vi "WHD_VEten_0.1.3_WS_BIDIR_Calibr.vi"() -> ()   [LabVIEW 2015]
uses:
  <vilib>/NI_Real-Time Target Support.lvlib
  <vilib>/rvi/interface/nirviReadWriteControl/nirviReadWriteControl.xnode
  <vilib>/rvi/interface/nirviMethod/nirviMethod.xnode
  <vilib>/rvi/interface/nirviOpenFPGA/nirviOpenFPGA.xnode
  <vilib>/rvi/interface/nirviCloseFPGA/nirviCloseFPGA.xnode
  <vilib>/userDefined/High Color/nirio_resource_hc.ctl
  <vilib>/rvi/errors/niLvFpgaMergeErrorWithErrorCode.vi
  <vilib>/Utility/file.llb/Write Delimited Spreadsheet (string).vi
  <vilib>/RTwatchdog.llb/Watchdog expiration actions.ctl
  <vilib>/nisyscfg/nisyscfg.lvlib
  AURA_Wheel/Json2Labv.lvlib
  AURA_Wheel/AuraWheelAPI/AuraWheel.lvlib
  <vilib>/rvi/errors/niLvFpgaAdjustHostInterfaceError.vi
  NiFpgaLv.dll
  <vilib>/Utility/error.llb/Error Cluster From Error Code.vi
  <vilib>/LabVIEW Targets/FPGA/cRIO/shared/nicrio_ModuleControls/nicrio_cRIO-9234_DataRatesRing2.ctl
  <vilib>/FPGAPlugInAG/cRIO-9031/niLvFpga_Run_cRIO-9031.vi
  <vilib>/FPGAPlugInAG/cRIO-9031/niLvFpga_ConfigureFifo_cRIO-9031.vi
  <vilib>/FPGAPlugInAG/cRIO-9031/niLvFpga_StartFifo_cRIO-9031.vi
  <vilib>/FPGAPlugInAG/cRIO-9031/niLvFpga_ReadFifo_cRIO-9031.vi
  <vilib>/FPGAPlugInAG/cRIO-9031/niLvFpga_StopFifo_cRIO-9031.vi
  <vilib>/FPGAPlugInAG/cRIO-9031/niLvFpga_Reset_cRIO-9031.vi
  <vilib>/measure/NI_MAPro.lvlib
  <vilib>/Analysis/NI_AALPro.lvlib
  <vilib>/measure/maspectr.llb/FFT Spectrum (Mag-Phase) for 1 Chan.vi
  <vilib>/Analysis/5stat.llb/RMS (DBL).vi
  <vilib>/measure/madcrms.llb/Basic Averaged DC-RMS for 1 Chan.vi
  FPGA Bitfiles/W&RDArabia_FPGATarget_FPGA8a2wsBIdirec_yJvL9yuTbZw.lvbitx
  <vilib>/FPGAPlugInAG/cRIO-9031/niLvFpga_Open_cRIO-9031.vi
  <vilib>/FPGAPlugInAG/cRIO-9031/niLvFpga_Close_cRIO-9031.vi
panel:
  in  "LR6 IP address":string="192.168.106.94"
  in  "Port LR6":u16=2001
  out "T fuera rango":bool
  in  "Frecuencia de muestreo (Hz)":dbl=25600.0
  in  "Escaneos de la FIFO por canal":u32=5000
  in  "Tiempo extra al detector de paso (s)":dbl=1.0
  in  "dt RMS":dbl=256.0
  in  "Frecuencia de muestreo y módulo CRIO":T1=2 items=["51.200 kS/s (NI 9234)"=1, "25.600 kS/s (NI 9234)"=2, "17.067 kS/s (NI 9234)"=3, "12.800 kS/s (NI 9234)"=4, "10.240 kS/s (NI 9234)"=5, "8.533 kS/s (NI 9234)"=6, "7.314 kS/s (NI 9234)"=7, "6.400 kS/s (NI 9234)"=8, "5.689 kS/s (NI 9234)"=9, "5.120 kS/s (NI 9234)"=10, "4.654 kS/s (NI 9234)"=11, "4.267 kS/s (NI 9234)"=12, "3.938 kS/s (NI 9234)"=13, "3.657 kS/s (NI 9234)"=14, "3.413 kS/s (NI 9234)"=15, "3.200 kS/s (NI 9234)"=16, "3.012 kS/s (NI 9234)"=17, "2.845 kS/s (NI 9234)"=18, "2.695 kS/s (NI 9234)"=19, "2.560 kS/s (NI 9234)"=20, "2.438 kS/s (NI 9234)"=21, "2.328 kS/s (NI 9234)"=22, "2.226 kS/s (NI 9234)"=23, "2.133 kS/s (NI 9234)"=24, "2.048 kS/s (NI 9234)"=25, "1.969 kS/s (NI 9234)"=26, "1.896 kS/s (NI 9234)"=27, "1.829 kS/s (NI 9234)"=28, "1.765 kS/s (NI 9234)"=29, "1.707 kS/s (NI 9234)"=30, "1.652 kS/s (NI 9234)"=31]
  in  "Puerto RFID":u16=2189
  in  "IP RFID":string="192.168.106.99"
  in  "Offset_rueda WS 2":fxp<+/-,24,-4>=0.004999998956918716 format="%.27g"
  in  "Count(mSec)":u32=2
  in  "RFID NEM on?":bool
  in  "RFID LR6 on?":bool
  in  "Canal cero WS1?":bool
  in  "Canal cero WS2":bool
  out "Inicio pasada 2":timestamp
  in  "Calibration":bool
  out "Direccion 0?":bool
  out "Boton Adquirir?":bool
  out "RuedaDetectada2?":bool=TRUE
  out "RuedaDetectada1?":bool=TRUE
  in  "Timeout ruedas":dbl
  in  "Borrar archivos\nadquisicion con error":bool
  in  "Able watchdog?":bool
  in  "Reset watchdog?":bool
  in  "Leer config RFID NEM":bool
  in  "bytes to read":i32
  in  "DeviceAddress":u8
  in  "timeout ms (60000)":i32
  in  "Max archivos":u32=2
  in  "Bytes libre despues de borrar":u32=2
  in  "Bytes min libre":u32=2
  in  "Nº de acelerómetros":i32
  in  "Nº inductivos":i32
  in  "Offset_rueda WS 1":fxp<+/-,24,-4>=0.004999998956918716 format="%.27g"
  out "TAGs_AURAwheel":string[][](array[string])
  out "Plataformas?":bool
  out "Nº Ejes":i32[](array[numeric])
  out "Nº UTs":i32
  out "it-read-LR6":i32[](array[numeric])
  out "it-LR6":i32
  out "RFID_LR6_Error":errorcluster
  out "Series_flota":string[](array[string])
  out "Tabla_flota":string[][](array[string])
  out "Puntos medios de las ventanas":dbl[][](array[numeric])
  out "configuration file path":path=path "c:/Parametros.cfg"
  in  "IP synchr":string
  out "data":cluster{"status":string}
  out "confRFID":path=path "c:/RFID/TAGS.csv"
  out "TAGS leidos":path=path "c:/RFID/TAGS.csv"
  in  "Use Aura?":bool
  in  "Parametros AuraWheel":string[](array[string])
  in  "Parámetros acelerómetros":dbl[](array[numeric])
  out "Fin":bool
  out "Contador":i32=1
  out "Path TEST":path=path "c:/TEST"
  out "Fallo fotocelula":bool
  out "Path_Borrar":path=path "c:/Trenes"
  out "Longitud de la unidad":dbl
  out "Aviso no detección":string
  out "Time to Acquire Block (ms)":i32
  out "Distancia de acelerómetros":dbl[](array[numeric])
  out "Block Size":u32
  out "Distancias generales":dbl[](array[numeric])
  in  "Reset del controlador":bool
  in  "Configuración":bool
  in  "Parar la aplicación":bool
  out "RFID":bool=TRUE
  out "date/time string":string
  out "Timeout ruedas":bool
  out "Tiempo":dbl
  out "Inicio pasada":timestamp
  out "Ultimo TEST":timestamp
  out "Fuente":bool=TRUE
  out "Estado":string
  out "RFID_ID":refnum<k5>
  out "DC OK":string
  out "Aviso temperatura":string
  in  "Tab Control":T2(tab)=enum."Datos adquisición"
  out "String":string
  out "V (m/s)":dbl
  out "Temperatura (ºC)":dbl
  out "Max RMS Ruedas":dbl[][](array[numeric])
  out "result":bool
  out "TAGs":string[](array[string])
  out "Parar":bool
  out "TAGs LR6":string[](array[string])
  out "TAGs HEX":string[](array[string])
  out "Waveform Graph 2":sgl[](graph)
  out "Waveform Graph":sgl[][](graph)
  out "Nombre de archivo":path[](array[path])
  out "Tiempo de paso (s)":dbl
  out "Tiempo extra de adquisición (s)":dbl
  out "Número de ejes detectados":i32
  out "Buffer Underflow":bool
  out "Buffer Overflow":bool
  out "Disco Duro Disponible (bytes)":i64
  out "created path":path
  out "Nº Ruedas 1":i32
  out "NºRuedas 2":i32
  out "deleted portion":sgl[](array[numeric])
  out "deleted portion 2":sgl[](array[numeric])
  out "Ejes_convoy":i32
  out "Archivo\nvalido?":bool
  out "Parámetros":bool=TRUE
  out "Distacias y medidas de dispositivos":bool=TRUE
  out "RFID_Error":errorcluster
  out "error FPGA":errorcluster
  out "error manipulacion archivos":errorcluster
  out "Unidades y ejes":bool=TRUE
  out "RFID":bool=TRUE
  out "error AURA":errorcluster
  out "Response headers":string
  out "Numeric 3":i32
  in  "Digital?":bool=TRUE
  out "Bucle Espera":i32
  out "Watchdog config":T3={"reset"=FALSE, "occurrence"=FALSE, "trigger protocol"=enum."active high", "trigger line"=enum."none", "disable watchdog on VI exit"=TRUE}
  out "error out":errorcluster
  in  "stop":bool
  in  "Tiempo de adquisicion":dbl=10.0
  in  "Adquirir":bool
  out "Waveform Graph 4":waveform(dbl)[](graph)
  out "Waveform Graph 3":cluster{"f0":dbl, "df":dbl, "magnitude":dbl[]}(graph)
  out "Chassis \nTemperature":i16
  out "Frecuencia de excitación\nVibrómetro  (Hz)":dbl
  out "Tiempo de paso (s) 2":dbl
  out "Nombre de archivo 2":path
  out "Buffer Overflow 2":bool
  out "Buffer Underflow 2":bool
  in  "Adquirir 2":bool
  in  "Nº del canal":i32
  in  "Parámetro de sensibilidad\n           (mV/g)":sgl=10.0
  in  "Aceleración del patrón (g RMS)":dbl=1.0
  in  "Frecuencia del patrón (Hz)":dbl=159.2
  # "Funciona?"
  # "Última detección de unidad"
  # "Error!!"
  # "Estado de la memoria"
  # "Cargar datos de configuración"
  # "Errores!!"
  # "WRD_MEX\nWRD_ZAR"
  # "0 tagMexInit\n1 tagMexFin\n\n0 tag1\n1 tag2"
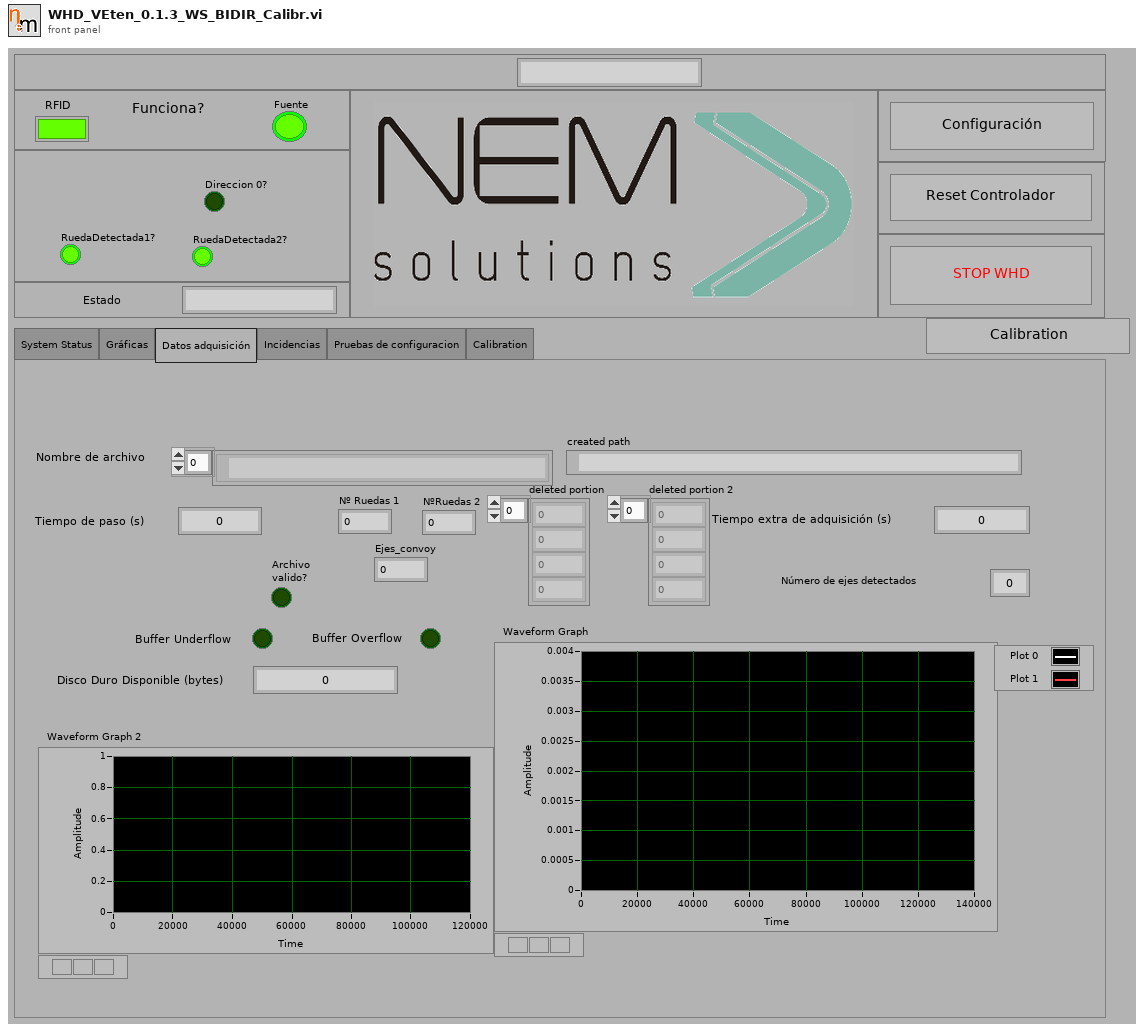
[diagram p1: front panel]
types:
  T1 = typedef "nicrio_cRIO-9234_DataRatesRing2.ctl" = u8
  T2 = enum32{"System Status", "Gráficas", "Datos adquisición", "Incidencias", "Pruebas de configuracion", "Calibration"}
  T3 = typedef "Watchdog expiration actions.ctl" = cluster{"reset":bool, "occurrence":bool, "trigger protocol":enum16{"active high", "active low", "open collector"}, "trigger line":enum16{"none", "line 0", "line 1", "line 2", "line 3", "line 4", "line 5", "line 6", "line 7", "SMB line 0"}, "disable watchdog on VI exit":bool}
  T4 = typedef "nirio_resource_hc.ctl" = tag
  T5 = enum16{"Standard", "Buffered", "CRLF", "Immediate"}
  T6 = enum16{"open", "replace", "create", "open or create", "replace or create", "replace or create with confirmation"}
  T7 = enum16{"big-endian, network order", "native, host order", "little-endian"}
  T8 = cluster{"error IO":errorcluster, bool[], u32[], string[], dbl[]}
  T9 = cluster{"g_ts":dbl, "p_sp":dbl, "p_tp":dbl, "p_tg":cluster{"tg_n":dbl, "tg_t":string}[], "p_ax":cluster{"ax_n":dbl, "ax_sp":dbl, "ax_wh":cluster{"wh_p":dbl, "wh_a1":dbl, "wh_a2":dbl, "wh_a3":dbl, "wh_a4":dbl}[]}[]}
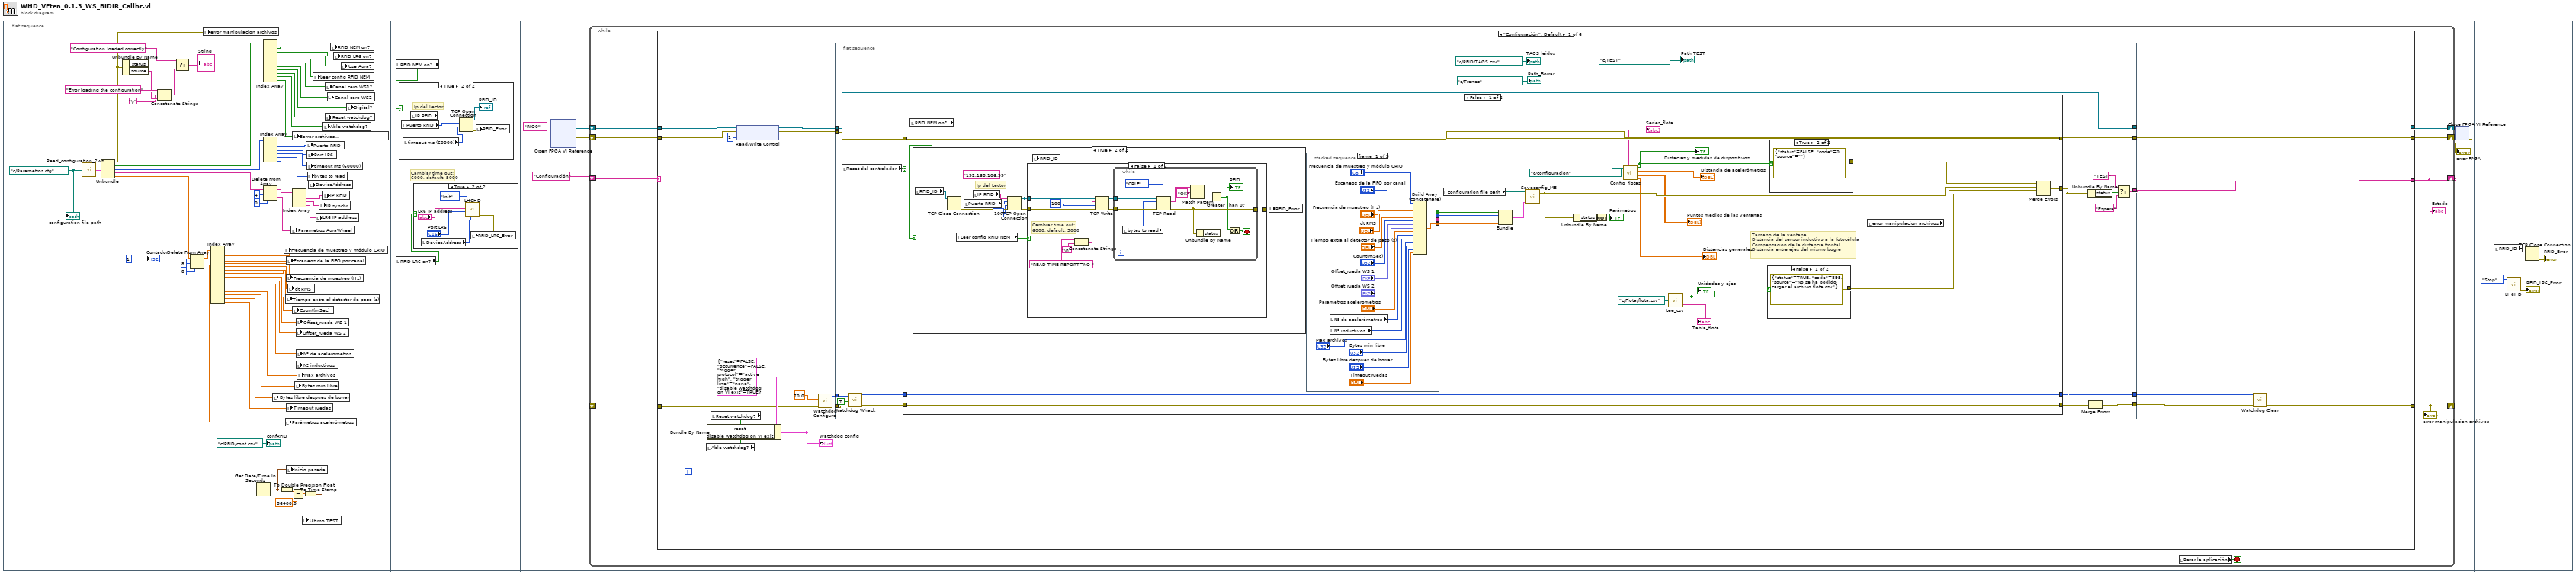
[diagram p0: block diagram]
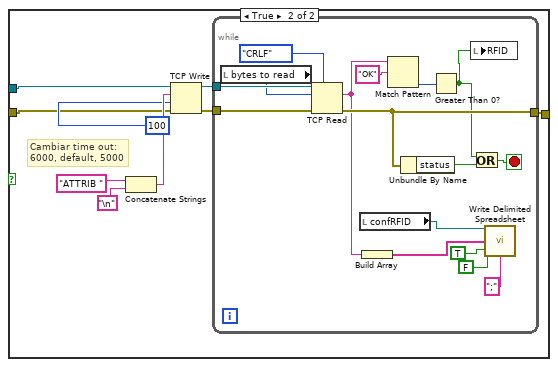
[diagram p5: hidden frame]
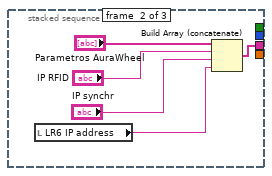
[diagram p6: hidden frame]
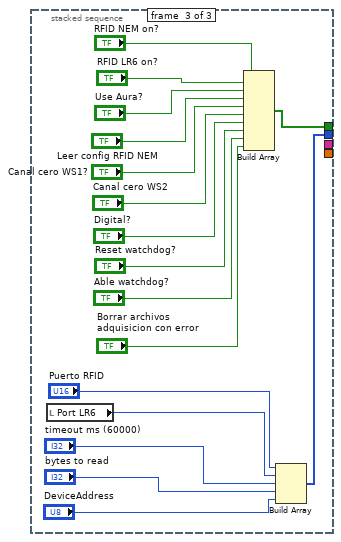
[diagram p7: hidden frame]
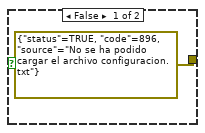
[diagram p8: hidden frame]
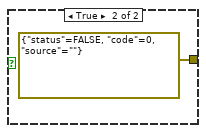
[diagram p9: hidden frame]
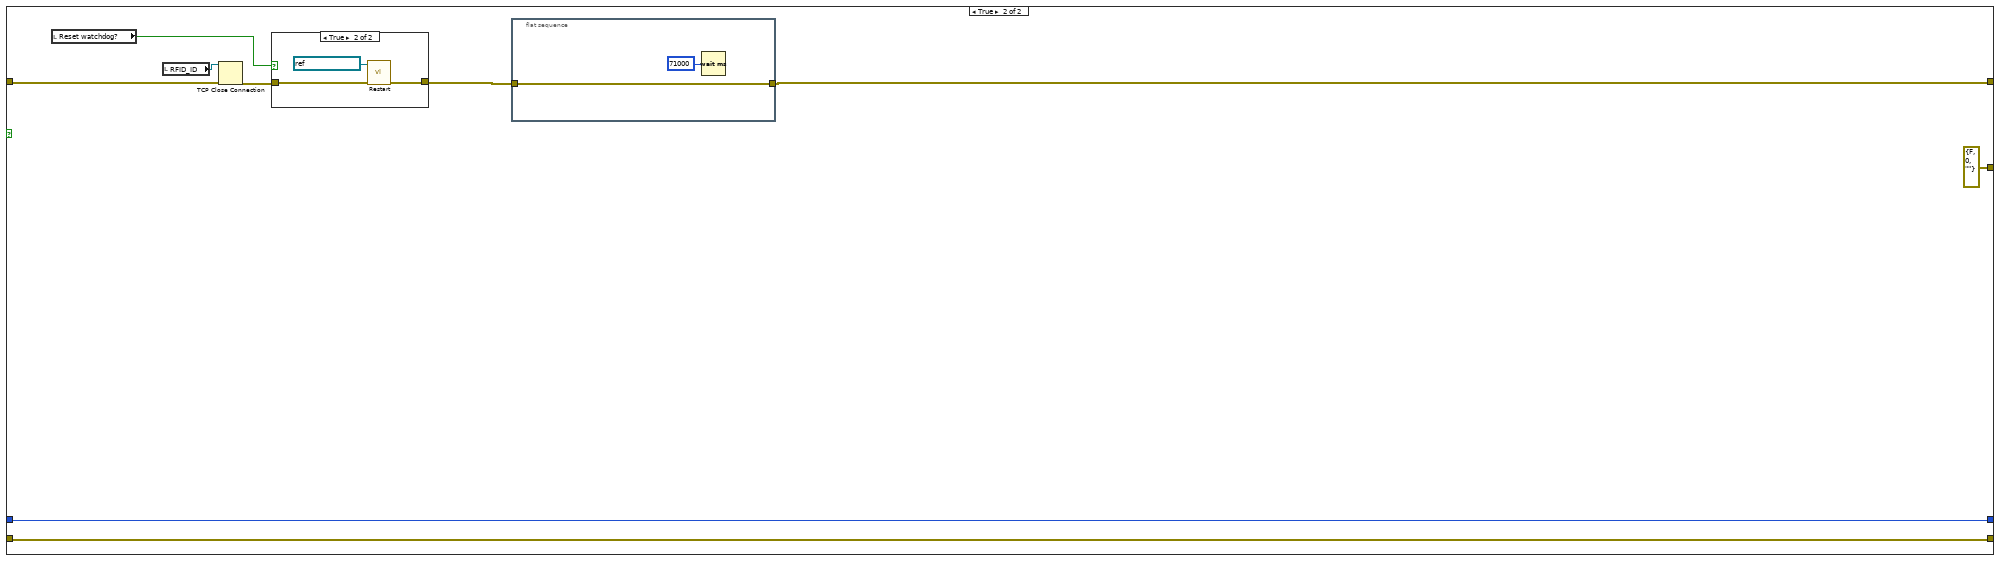
[diagram p10: hidden frame]
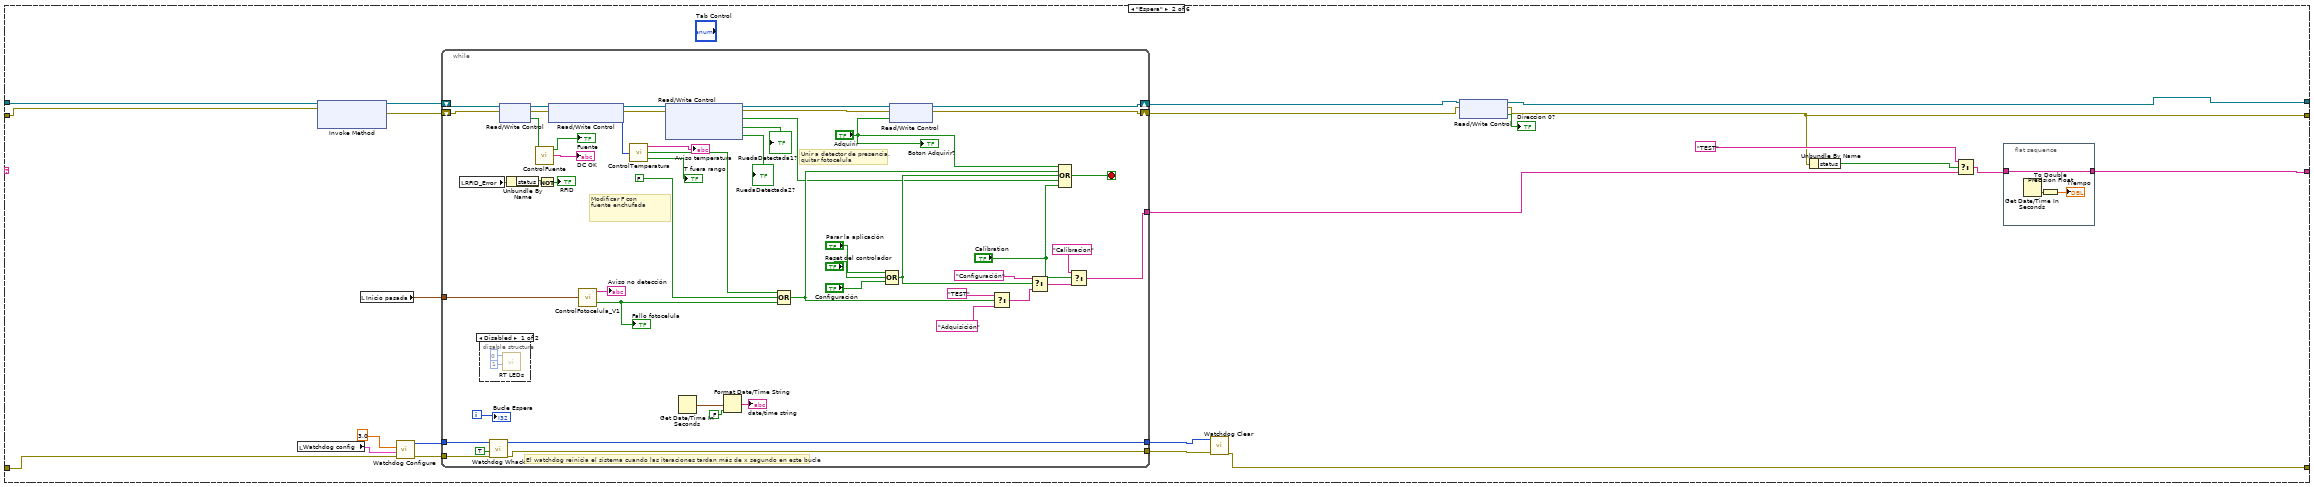
[diagram p12: hidden frame]
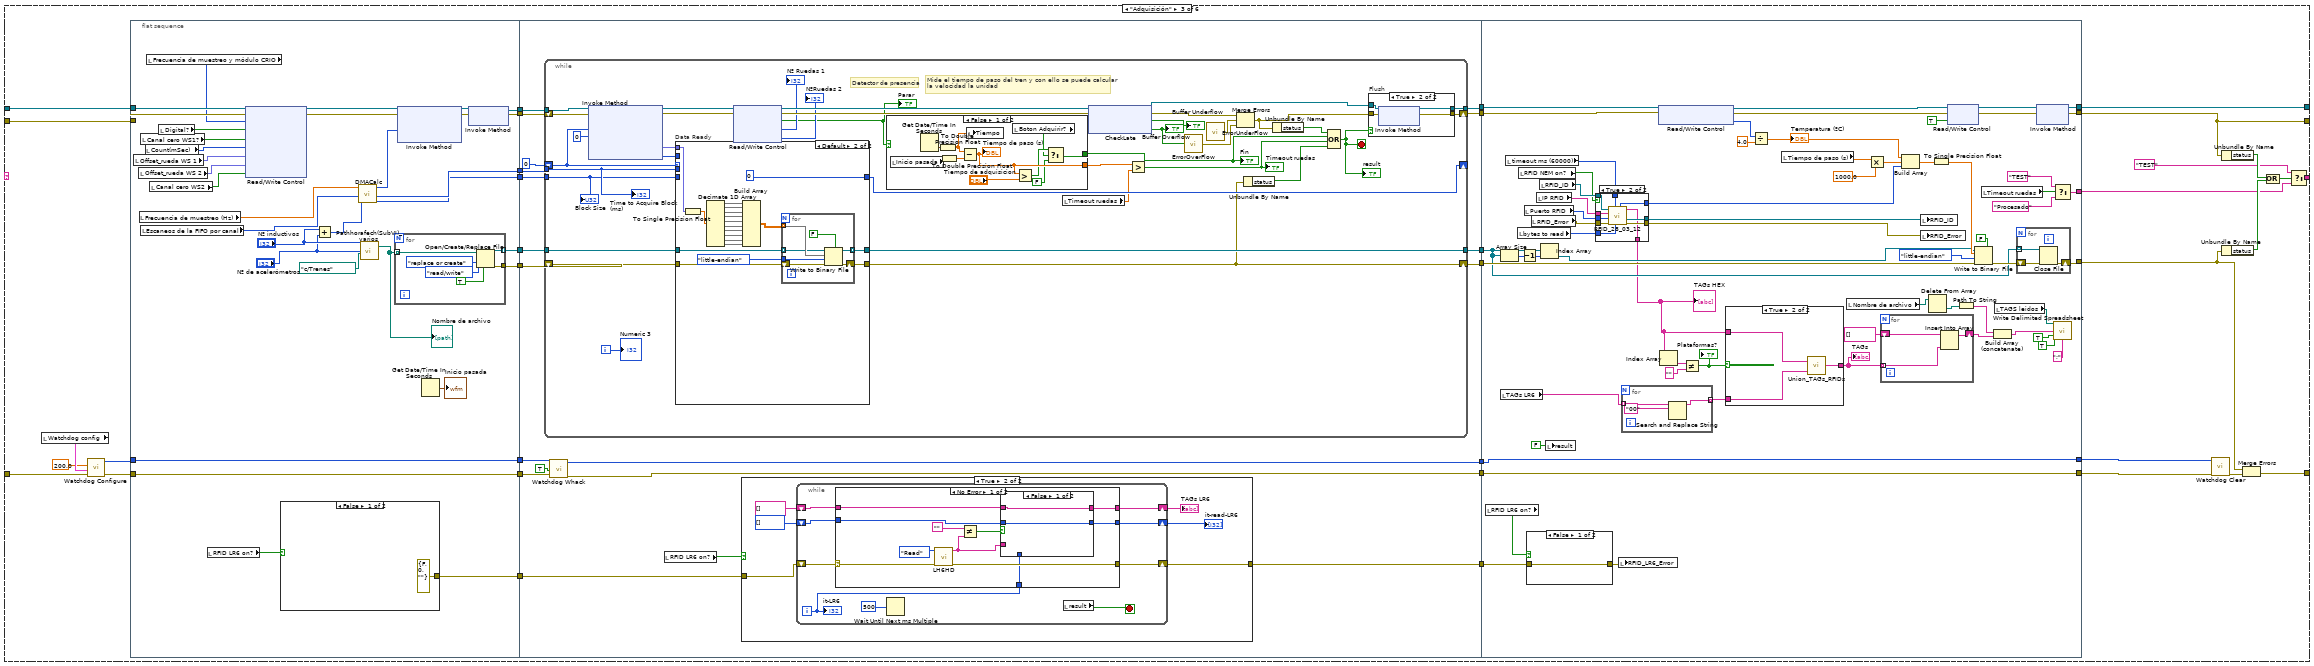
[diagram p14: hidden frame]
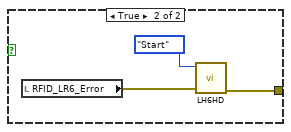
[diagram p15: hidden frame]
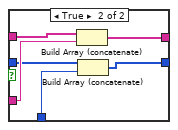
[diagram p17: hidden frame]
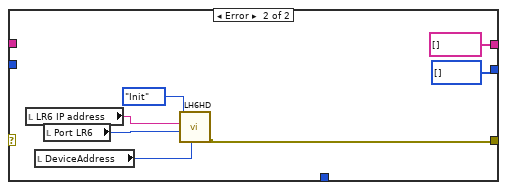
[diagram p18: hidden frame]
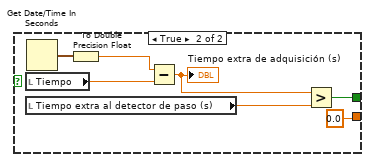
[diagram p19: hidden frame]
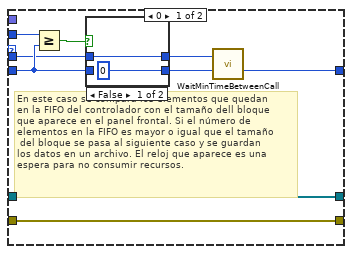
[diagram p20: hidden frame]
diagram:
  n1 = flat-sequence {
    frame #0 {
      w46 = path "c:/Parametros.cfg" ("configuration file path")
      n2 = call "Read_configuration_2ws.vi"("configuration file path"=w46) -> ("output cluster"=w45:T8)
      n3 = Unbundle(w45) -> ("error IO"=w8:errorcluster, w49:bool[], w48:u32[], w37:string[], w43:dbl[])
      n4 = Unbundle By Name(w8) -> ("status"=w7:bool, "source"=w4:string)
      n5 = Concatenate Strings("Error loading the configuration", "\r", w4) -> (w2:string)
      n6 = Select(t="Configuration loaded correctly", s=w7, f=w2) -> (s? t:f=→"String":string)
      n7 = Delete From Array(array=w43, length=8, index=8) -> (deleted portion=w39:dbl[], array with subset deleted=w42:dbl[])
      n8 = local write "error manipulacion archivos"(w8) -> ()
      n9 = Index Array(array=w42) -> (element #1=w56:dbl, element #2=w55:dbl, element #3=w54:dbl, element #4=w53:dbl, element #5=w52:dbl, element #6=w27:dbl, element #7=w26:dbl, element #8=w9:dbl, element #9=w25:dbl, element #10=w24:dbl, element #11=w23:dbl, element #12=w22:dbl, element #13=w21:dbl, element #14=w10:dbl)  [unwired: 14 in]
      n10 = Get Date/Time In Seconds() -> (seconds since 1Jan1904=w58:timestamp)
      n11 = Index Array(array=w49) -> (element #1=w51:bool, element #2=w50:bool, element #3=w38:bool, element #4=w17:bool, element #5=w16:bool, element #6=w15:bool, element #7=w14:bool, element #8=w13:bool, element #9=w12:bool, element #10=w11:bool)  [unwired: 10 in]
      n12 = Index Array(array=w48) -> (element #1=w44:u32, element #2=w28:u32, element #3=w20:u32, element #4=w19:u32, element #5=w18:u32)  [unwired: 5 in]
      n13 = Delete From Array(array=w37, length=4, index=0) -> (deleted portion=w31:string[], array with subset deleted=w36:string[])
      n14 = local write "Bytes libre despues de borrar"(w21) -> ()
      n15 = To Double Precision Float(number=w58) -> (double precision float=w60:dbl)
      n16 = local write "Frecuencia de muestreo y módulo CRIO"(w56) -> ()
      n17 = local write "Parámetros acelerómetros"(w39) -> ()
      n18 = local write "Tiempo extra al detector de paso (s)"(w52) -> ()
      n19 = local write "Frecuencia de muestreo (Hz)"(w54) -> ()
      n20 = local write "Timeout ruedas"(w10) -> ()
      n21 = local write "Escaneos de la FIFO por canal"(w55) -> ()
      n22 = local write "Inicio pasada"(w58) -> ()
      n23 = local write "dt RMS"(w53) -> ()
      n24 = local write "Parametros AuraWheel"(w31) -> ()
      n25 = Subtract(x=w60, y=86400.0) -> (x-y=w59:dbl)
      n26 = local write "Borrar archivos\nadquisicion con error"(w11) -> ()
      n27 = Index Array(array=w36) -> (element #1=w30:string, element #2=w32:string, element #3=w29:string)  [unwired: 3 in]
      n28 = local write "Count(mSec)"(w27) -> ()
      n29 = local write "Bytes min libre"(w22) -> ()
      n30 = local write "Offset_rueda WS 2"(w9) -> ()
      n31 = local write "Offset_rueda WS 1"(w26) -> ()
      n32 = local write "Nº de acelerómetros"(w25) -> ()
      n33 = local write "Nº inductivos"(w24) -> ()
      n34 = local write "Max archivos"(w23) -> ()
      n35 = To Time Stamp(1:w59) -> (0:w57:timestamp)
      n36 = local write "Ultimo TEST"(w57) -> ()
      n37 = local write "Puerto RFID"(w44) -> ()
      n38 = local write "Port LR6"(w28) -> ()
      n39 = local write "timeout ms (60000)"(w20) -> ()
      n40 = local write "bytes to read"(w19) -> ()
      n41 = local write "DeviceAddress"(w18) -> ()
      n42 = local write "Leer config RFID NEM"(w17) -> ()
      n43 = local write "LR6 IP address"(w29) -> ()
      n44 = local write "IP synchr"(w32) -> ()
      n45 = local write "IP RFID"(w30) -> ()
      n46 = local write "Able watchdog?"(w12) -> ()
      n47 = local write "Reset watchdog?"(w13) -> ()
      n48 = local write "Canal cero WS1?"(w16) -> ()
      n49 = local write "Canal cero WS2"(w15) -> ()
      n50 = local write "RFID NEM on?"(w51) -> ()
      n51 = local write "RFID LR6 on?"(w50) -> ()
      n52 = local write "Use Aura?"(w38) -> ()
      n53 = local write "Digital?"(w14) -> ()
      "Contador" <- 1
      "confRFID" <- path "c:/RFID/conf.csv" ("file path (use dialog)")
      "configuration file path" <- w46
    }
    frame #1 {
      # "Cambiar time out:\n6000, default, 5000"
      n54 = local read "RFID NEM on?"() -> (w63:bool)
      n55 = local read "RFID LR6 on?"() -> (w62:bool)
      n56 = case shown="True" w63 {
        frame False {
        }
        frame True {
          # "Ip del Lector"
          n57 = local read "Puerto RFID"() -> (w71:u16)
          n58 = local read "timeout ms (60000)"() -> (w69:i32)
          n59 = local read "IP RFID"() -> (w72:string)
          n60 = TCP Open Connection(address=w72, remote port or service name=w71, timeout ms (60000)=w69) -> (connection ID=→"RFID_ID":refnum<k5>, error out=w70:errorcluster)  [unwired: 1 in, 1 out]
          n61 = local write "RFID_Error"(w70) -> ()
        }
      }
      n62 = case shown="True" w62 {
        frame False {
        }
        frame True {
          n63 = local read "DeviceAddress"() -> (w64:u8)
          n64 = call "LH6HD.vi"("DeviceAddress"=w64, "Reader Port"="Port LR6", "IP Address"="LR6 IP address", "Action"=enum16{"Init", "Start", "Read", "Stop", "Exit"}."Init") -> ("error out"=w68:errorcluster)  [unwired: 6 in, 1 out]
          n65 = local write "RFID_LR6_Error"(w68) -> ()
        }
      }
    }
    frame #2 {
      n66 = xnode "Open FPGA VI Reference"("resource name"=T4 "RIO0") -> ("FPGA VI Reference Out"=w80:refnum<k20>, "error out"=w79:errorcluster)  [unwired: 1 in]
      n67 = while {
        shift-right: [w81] -> _
        shift-left: "Configuración" -> [w89]
        shift-right: [w83] -> w76
        shift-left: w80 -> [w88]
        shift-right: [w82] -> w75
        shift-left: w79 -> [w87]
        shift-right: [w86] -> _
        shift-left: _ -> [w85]
        stop <- w84 stop-if-true
        n68 = case shown="\"Configuración\", Default" w89 {
          tunnel: [w95 w279 w358 w689 w930 _] -> w81
          tunnel: [w107 w267 w372 w697 w929 _] -> w83
          tunnel: [w108 w266 w373 w684 w927 _] -> w82
          tunnel: w88 -> [w100 w284 w380 w697 w929 w1002]
          tunnel: w87 -> [w98 w282 w379 w684 w928 w1001]
          tunnel: [w104 w273 w370 w687 w917 _] -> w86
          tunnel: w85 -> [w94 w278 w354 w683 w922 _]
          frame "Configuración", Default {
            n69 = local read "Able watchdog?"() -> (w101:bool)
            n70 = local read "Reset watchdog?"() -> (w102:bool)
            n71 = Bundle By Name(cluster=T3 {"reset"=FALSE, "occurrence"=FALSE, "trigger protocol"=enum."active high", "trigger line"=enum."none", "disable watchdog on VI exit"=TRUE} ("expiration actions"), "reset"=w102, "disable watchdog on VI exit"=w101) -> (w93:T3)
            "Watchdog config" <- w93
            n72 = xnode "Read/Write Control"("FPGA VI Reference In"=w100, "error in"=w98, "Cycles to Filter"=u16 1) -> ("FPGA VI Reference Out"=w99:refnum<k20>, "error out"=w97:errorcluster)
            n73 = call <vilib>:"Watchdog Configure.vi"("error in (no error)"=w94, "expiration actions"=w93, "timeout (1 sec)"=70.0) -> ("error out"=w90:errorcluster, "watchdogID"=w91:u64)  [unwired: 1 in, 2 out]
            n74 = flat-sequence {
              tunnel: [w119] -> w108
              tunnel: [w127] -> w95
              tunnel: w99 -> [w120]
              tunnel: [w120] -> w107
              tunnel: [w122] -> w105
              tunnel: w97 -> [w117]
              tunnel: [w114] -> w106
              tunnel: w91 -> [w110]
              tunnel: w90 -> [w109]
              frame #0 {
                n75 = local read "Reset del controlador"() -> (w116:bool)
                n76 = call <vilib>:"Watchdog Whack.vi"("error in (no error)"=w109, "reset watchdog after expire? (F)"=TRUE, "watchdogID in"=w110) -> ("error out"=w112:errorcluster, "watchdogID out"=w113:u64)  [unwired: 2 in, 1 out]
                n77 = case shown="False" w116 {
                  tunnel: w117 -> [w154 w257]
                  tunnel: [w154 w256] -> w119
                  tunnel: [w140 errorcluster {"status"=FALSE, "code"=0, "source"=""} ("error IO")] -> w118
                  tunnel: [w132 w255] -> w114
                  tunnel: w113 -> [w132 w255]
                  tunnel: w112 -> [w131 w254]
                  tunnel: [w131 w254] -> w111
                  frame False {
                    # "Tamaño de la ventana\nDistancia del sensor inductivo a la fotocélula\nCompensación de la distancia frontal\nDistancia entre ejes del mismo bogie"
                    n78 = local read "RFID NEM on?"() -> (w130:bool)
                    n79 = case shown="True" w130 {
                      frame False {
                      }
                      frame True {
                        (unwired) "192.168.106.99" ("address")
                        # "Ip del Lector"
                        n80 = local read "RFID_ID"() -> (w162:refnum<k5>)
                        n81 = TCP Close Connection(connection ID=w162) -> (error out=w163:errorcluster)  [unwired: 2 in, 1 out]
                        n82 = local read "Leer config RFID NEM"() -> (w155:bool)
                        n83 = local read "Puerto RFID"() -> (w160:u16)
                        n84 = local read "IP RFID"() -> (w159:string)
                        n85 = TCP Open Connection(address=w159, remote port or service name=w160, timeout ms (60000)=100, error in (no error)=w163) -> (connection ID=w161:refnum<k5>, error out=w156:errorcluster)  [unwired: 1 out]
                        n86 = case shown="False" w155 {
                          tunnel: w161 -> [w172 w186]
                          tunnel: [w170 w184] -> w157
                          tunnel: w156 -> [w167 w185]
                          frame False {
                            # "Cambiar time out:\n6000, default, 5000"
                            n87 = Concatenate Strings("READ TIME REPORT=NO " ("data in"), "\n") -> (w164:string)
                            n88 = TCP Write(connection ID=w172, data in=w164, error in (no error)=w167, 9:100 ("timeout ms (25000)")) -> (connection ID out=w168:refnum<k5>, error out=w169:errorcluster)  [unwired: 1 out]
                            n89 = while {
                              tunnel: w169 -> [w182]
                              tunnel: w168 -> [w181]
                              tunnel: [w180] -> w170
                              stop <- w177 stop-if-true
                              n90 = local read "bytes to read"() -> (w173:i32)
                              n91 = TCP Read(connection ID=w181, bytes to read=w173, error in (no error)=w182, 7:T5."CRLF" ("mode (standard)")) -> (data out=w175:string, error out=w180:errorcluster)  [unwired: 1 in, 1 out]
                              n92 = Match Pattern(string=w175, regular expression="OK") -> (offset past match=w178:i32)  [unwired: 4 out]
                              n93 = Unbundle By Name(w180) -> ("status"=w176:bool)
                              n94 = Greater Than 0?(x=w178) -> (x > 0?=w174:bool)
                              "RFID" <- w174
                              n95 = Or(x=w174, y=w176) -> (x .or. y?=w177:bool)
                            }
                          }
                          frame True {
                            # "Cambiar time out:\n6000, default, 5000"
                            n96 = Concatenate Strings("ATTRIB " ("data in"), "\n") -> (w192:string)
                            n97 = TCP Write(connection ID=w186, data in=w192, error in (no error)=w185, 9:100 ("timeout ms (25000)")) -> (connection ID out=w189:refnum<k5>, error out=w188:errorcluster)  [unwired: 1 out]
                            n98 = while {
                              tunnel: w188 -> [w207]
                              tunnel: w189 -> [w206]
                              tunnel: [w205] -> w184
                              stop <- w202 stop-if-true
                              n99 = local read "bytes to read"() -> (w193:i32)
                              n100 = TCP Read(connection ID=w206, bytes to read=w193, error in (no error)=w207, 7:T5."CRLF" ("mode (standard)")) -> (data out=w196:string, error out=w205:errorcluster)  [unwired: 1 in, 1 out]
                              n101 = local read "confRFID"() -> (w195:path)
                              n102 = Build Array(w196) -> (w194:string[])
                              n103 = Match Pattern(string=w196, regular expression="OK") -> (offset past match=w203:i32)  [unwired: 4 out]
                              n104 = Unbundle By Name(w205) -> ("status"=w201:bool)
                              n105 = Greater Than 0?(x=w203) -> (x > 0?=w200:bool)
                              n106 = local write "RFID"(w200) -> ()
                              n107 = Or(x=w200, y=w201) -> (x .or. y?=w202:bool)
                              n108 = call-poly <vilib>:"Write Delimited Spreadsheet.vi"("file path (dialog if empty)"=w195, "1D data"=w194, "append to file? (F)"=FALSE ("transpose? (no:F)"), "transpose? (F)"=TRUE ("append to file? (new file:F)"), "delimiter (\\t)"=";" ("delimiter (\\t)")) -> ()  [unwired: 9 in, 2 out]
                            }
                          }
                        }
                        n109 = local write "RFID_ID"(w161) -> ()
                        n110 = local write "RFID_Error"(w157) -> ()
                      }
                    }
                    n111 = stacked-sequence {
                      tunnel: [w220 _ _] -> w144
                      tunnel: [_ w229 _] -> w143
                      tunnel: [_ _ w243] -> w145
                      tunnel: [_ _ w242] -> w146
                      frame #0 {
                        n112 = local read "Nº de acelerómetros"() -> (w214:i32)
                        n113 = local read "Nº inductivos"() -> (w213:i32)
                        n114 = Build Array (concatenate)("Frecuencia de muestreo y módulo CRIO", "Escaneos de la FIFO por canal", "Frecuencia de muestreo (Hz)", "dt RMS", "Tiempo extra al detector de paso (s)", "Count(mSec)", "Offset_rueda WS 1", "Offset_rueda WS 2", "Parámetros acelerómetros", w214, w213, "Max archivos", "Bytes min libre", "Bytes libre despues de borrar", "Timeout ruedas") -> (w220:dbl[])
                      }
                      frame #1 {
                        n115 = local read "LR6 IP address"() -> (w225:string)
                        n116 = Build Array (concatenate)("Parametros AuraWheel", "IP RFID", "IP synchr", w225) -> (w229:string[])
                      }
                      frame #2 {
                        n117 = local read "Port LR6"() -> (w239:u16)
                        n118 = Build Array("RFID NEM on?", "RFID LR6 on?", "Use Aura?", "Leer config RFID NEM", "Canal cero WS1?", "Canal cero WS2", "Digital?", "Reset watchdog?", "Able watchdog?", "Borrar archivos\nadquisicion con error") -> (w242:bool[])
                        n119 = Build Array("Puerto RFID", w239, "timeout ms (60000)", "bytes to read", "DeviceAddress") -> (w243:i32[])
                      }
                    }
                    n120 = local read "configuration file path"() -> (w141:path)
                    n121 = Bundle(w146, w145, w143, w144) -> (w142:cluster{bool[], i32[], string[], dbl[]})  [unwired: 1 in]
                    n122 = call "Saveconfig_MB.vi"("configuration file path"=w141, "Configuracion"=w142) -> ("error out"=w149:errorcluster)  [unwired: 4 in]
                    n123 = Unbundle By Name(w149) -> ("status"=w150:bool)
                    n124 = Not(x=w150) -> (.not. x?=→"Parámetros":bool)
                    n125 = call "Config_flotas.vi"("file path (dialog if empty)"=path "c:/configuracion") -> ("Distancias generales"=→"Distancias generales":dbl[], "Puntos medios de las ventanas"=→"Puntos medios de las ventanas":dbl[][], "Distancia de acelerómetros"=→"Distancia de acelerómetros":dbl[], "Distacias y medidas de dispositivos"=w139:bool, "Series_flota"=→"Series_flota":string[])  [unwired: 3 in]
                    "Distacias y medidas de dispositivos" <- w139
                    n126 = call "Lee_csv.vi"("Path"=path "c:/Flota/flota.csv") -> ("Tabla_flota"=→"Tabla_flota":string[][], "Lectura_OK?"=w136:bool)
                    "Unidades y ejes" <- w136
                    n127 = case shown="False" w136 {
                      tunnel: [errorcluster {"status"=TRUE, "code"=895, "source"="No se ha podido cargar el archivo flota.csv"} ("error out") errorcluster {"status"=FALSE, "code"=0, "source"=""} ("error out")] -> w147
                      frame False {
                      }
                      frame True {
                      }
                    }
                    n128 = case shown="True" w139 {
                      tunnel: [errorcluster {"status"=TRUE, "code"=896, "source"="No se ha podido cargar el archivo configuracion.txt"} ("error out") errorcluster {"status"=FALSE, "code"=0, "source"=""} ("error out")] -> w152
                      frame False {
                      }
                      frame True {
                      }
                    }
                    n129 = local read "error manipulacion archivos"() -> (w148:errorcluster)
                    n130 = Merge Errors(w152, w149, w148, w147) -> (w140:errorcluster)
                  }
                  frame True {
                    n131 = local read "Reset watchdog?"() -> (w251:bool)
                    n132 = local read "RFID_ID"() -> (w259:refnum<k5>)
                    n133 = TCP Close Connection(connection ID=w259, error in (no error)=w257) -> (error out=w253:errorcluster)  [unwired: 2 out]
                    n134 = case shown="True" w251 {
                      tunnel: w253 -> [w260 w263]
                      tunnel: [w260 w262] -> w252
                      frame False {
                      }
                      frame True {
                        n135 = call <vilib>:"Restart.vi"("error in (no error)"=w263, "Session in"=refnum<k21> "localhost") -> ("error out"=w262:errorcluster)  [unwired: 7 in, 2 out]
                      }
                    }
                    n136 = flat-sequence {
                      tunnel: [w265] -> w256
                      tunnel: w252 -> [w265]
                      frame #0 {
                        n137 = Wait (ms)(milliseconds to wait=u32 71000) -> ()  [unwired: 1 out]
                      }
                    }
                  }
                }
                n138 = Unbundle By Name(w118) -> ("status"=w128:bool)
                n139 = Merge Errors(w118, w111) -> (w122:errorcluster)
                n140 = Select(t="TEST", s=w128, f="Espera") -> (s? t:f=w127:string)
                "Path_Borrar" <- path "c:/Trenes" ("file path (use dialog)")
                "Path TEST" <- path "c:/TEST" ("file path (use dialog)")
                "TAGS leidos" <- path "c:/RFID/TAGS.csv" ("file path (use dialog)")
              }
            }
            n141 = call <vilib>:"Watchdog Clear.vi"("error in (no error)"=w105, "watchdogID in"=w106) -> ("error out"=w104:errorcluster)  [unwired: 5 in]
          }
          frame "Espera" {
            n142 = local read "Watchdog config"() -> (w272:T3)
            n143 = xnode "Invoke Method"("FPGA VI Reference In"=w284, "error in"=w282) -> ("FPGA VI Reference Out"=w283:refnum<k20>, "error out"=w281:errorcluster)  [unwired: 1 in]
            n144 = local read "Inicio pasada"() -> (w288:timestamp)
            n145 = call <vilib>:"Watchdog Configure.vi"("error in (no error)"=w278, "expiration actions"=w272, "timeout (1 sec)"=3.0) -> ("error out"=w277:errorcluster, "watchdogID"=w276:u64)  [unwired: 1 in, 2 out]
            n146 = while {
              tunnel: [w294] -> w287
              shift-right: [w304] -> w268
              shift-left: w283 -> [w317]
              shift-right: [w303] -> w269
              shift-left: w281 -> [w316]
              tunnel: w288 -> [w320]
              tunnel: w277 -> [w301]
              tunnel: w276 -> [w302]
              tunnel: [w300] -> w275
              tunnel: [w299] -> w274
              i -> [w297]
              stop <- w292 stop-if-true
              # "Modificar F con\nfuente enchufada"
              # "Unir a detector de presencia,\nquitar fotocelula"
              # "El watchdog reinicia el sistema cuando las iteraciones tardan más de x segundo en este bucle"
              n147 = local read "RFID_Error"() -> (w323:errorcluster)
              n148 = disable-structure shown="Disabled" {
                frame Disabled {
                  n149 = call <vilib>:"RT LEDs.vi"("State"=1, "LED Num"=0) -> ()  [unwired: 1 in, 5 out]
                }
                frame Enabled {
                }
              }
              n150 = call <vilib>:"Watchdog Whack.vi"("error in (no error)"=w301, "reset watchdog after expire? (F)"=TRUE, "watchdogID in"=w302) -> ("error out"=w299:errorcluster, "watchdogID out"=w300:u64)  [unwired: 2 in, 1 out]
              n151 = xnode "Read/Write Control"("FPGA VI Reference In"=w317, "error in"=w316) -> ("FPGA VI Reference Out"=w334:refnum<k20>, "error out"=w333:errorcluster, "DC OK"=w338:bool)
              n152 = Unbundle By Name(w323) -> ("status"=w321:bool)
              n153 = call "ControlFuente.vi"("DC OK 3"=w338) -> ("DC OK 2"=→"Fuente":bool, "DC OK"=→"DC OK":string)  [unwired: 1 out]
              n154 = Not(x=w321) -> (.not. x?=→"RFID":bool)
              n155 = xnode "Read/Write Control"("FPGA VI Reference In"=w334, "error in"=w333) -> ("FPGA VI Reference Out"=w329:refnum<k20>, "error out"=w328:errorcluster, "Chassis Temperature"=w336:i16)
              n156 = call "ControlFotocelula_V1.vi"("Tiempo de entrada a espera"=w320) -> ("Aviso no detección"=→"Aviso no detección":string, "Boolean"=w326:bool)
              "Fallo fotocelula" <- w326
              n157 = call "ControlTemperatura.vi"("Chassis Temperature"=w336) -> ("Aviso temperatura"=→"Aviso temperatura":string, "Boolean"=w330:bool, "T fuera rango"=→"T fuera rango":bool)
              n158 = xnode "Read/Write Control"("FPGA VI Reference In"=w329, "error in"=w328) -> ("FPGA VI Reference Out"=w319:refnum<k20>, "error out"=w318:errorcluster, "Detector de presencia"=w311:bool, "RuedaDetectada1?"=→"RuedaDetectada1?":bool, "RuedaDetectada2?"=→"RuedaDetectada2?":bool)
              n159 = Get Date/Time In Seconds() -> (seconds since 1Jan1904=w313:timestamp)
              n160 = Format Date/Time String(seconds (now)=w313, UTC format=FALSE) -> (date/time string=→"date/time string":string)  [unwired: 1 in]
              n161 = Compound Arithmetic op=OR(w330, FALSE ("value"), w326) -> (w327:bool)
              n162 = Compound Arithmetic op=OR("Parar la aplicación", "Reset del controlador", "Configuración") -> (w324:bool)
              n163 = xnode "Read/Write Control"("FPGA VI Reference In"=w319, "error in"=w318, "Fotocélula"="Adquirir") -> ("FPGA VI Reference Out"=w304:refnum<k20>, "error out"=w303:errorcluster)
              n164 = Select(t="TEST", s=w327, f="Adquisición") -> (s? t:f=w339:string)
              n165 = Select(t="Configuración", s=w324, f=w339) -> (s? t:f=w296:string)
              n166 = Compound Arithmetic op=OR("Adquirir", w327, w324, w311, "Calibration") -> (w292:bool)
              n167 = Select(t="Calibracion", s="Calibration", f=w296) -> (s? t:f=w294:string)
              "Bucle Espera" <- w297
              "Boton Adquirir?" <- "Adquirir"
            }
            n168 = call <vilib>:"Watchdog Clear.vi"("error in (no error)"=w274, "watchdogID in"=w275) -> ("error out"=w273:errorcluster)  [unwired: 5 in]
            n169 = xnode "Read/Write Control"("FPGA VI Reference In"=w268, "error in"=w269) -> ("FPGA VI Reference Out"=w267:refnum<k20>, "error out"=w266:errorcluster, "Direccion 0?"=→"Direccion 0?":bool)
            n170 = Unbundle By Name(w266) -> ("status"=w286:bool)
            n171 = Select(t="TEST", s=w286, f=w287) -> (s? t:f=w280:string)
            n172 = flat-sequence {
              tunnel: [w290] -> w279
              tunnel: w280 -> [w290]
              frame #0 {
                n173 = Get Date/Time In Seconds() -> (seconds since 1Jan1904=w291:timestamp)
                n174 = To Double Precision Float(number=w291) -> (double precision float=→"Tiempo":dbl)
              }
            }
          }
          frame "Adquisición" {
            n175 = local read "Watchdog config"() -> (w355:T3)
            n176 = call <vilib>:"Watchdog Configure.vi"("error in (no error)"=w354, "expiration actions"=w355, "timeout (1 sec)"=200.0) -> ("error out"=w352:errorcluster, "watchdogID"=w353:u64)  [unwired: 1 in, 2 out]
            n177 = flat-sequence {
              tunnel: w379 -> [w408]
              tunnel: w380 -> [w409]
              tunnel: [w407] -> w369
              tunnel: [w406] -> w368
              tunnel: [w405] -> w367
              tunnel: [w404] -> w366
              tunnel: [w403] -> w365
              tunnel: [w402] -> w364
              tunnel: [w391] -> w357
              tunnel: w353 -> [w390]
              tunnel: w352 -> [w389]
              tunnel: [w390] -> w351
              tunnel: [w389] -> w350
              tunnel: [w424] -> w378
              tunnel: [w441] -> w377
              tunnel: [w440] -> w376
              tunnel: [w439] -> w375
              tunnel: [w432] -> w374
              tunnel: w369 -> [w438]
              tunnel: w368 -> [w437]
              tunnel: w367 -> [w436]
              tunnel: w366 -> [w435]
              tunnel: w365 -> [w434]
              tunnel: w364 -> [w433]
              tunnel: w357 -> [w430]
              tunnel: [w429] -> w356
              tunnel: w351 -> [w428]
              tunnel: w350 -> [w427]
              tunnel: [w425] -> w349
              tunnel: w378 -> [w589]
              tunnel: w377 -> [w584]
              tunnel: w376 -> [w583]
              tunnel: w375 -> [w605]
              tunnel: [w635] -> w361
              tunnel: w374 -> [w637]
              tunnel: [w621] -> w371
              tunnel: [w622] -> w373
              tunnel: [w623] -> w372
              tunnel: w356 -> [w599]
              tunnel: w349 -> [w590]
              tunnel: [w590] -> w347
              tunnel: [w589] -> w346
              frame #0 {
                n178 = local read "Offset_rueda WS 1"() -> (w382:fxp<+/-,24,-4>)
                n179 = local read "Offset_rueda WS 2"() -> (w383:fxp<+/-,24,-4>)
                n180 = local read "Frecuencia de muestreo (Hz)"() -> (w400:dbl)
                n181 = local read "Escaneos de la FIFO por canal"() -> (w388:u32)
                n182 = local read "Canal cero WS1?"() -> (w393:bool)
                n183 = local read "Count(mSec)"() -> (w392:u32)
                n184 = local read "Frecuencia de muestreo y módulo CRIO"() -> (w395:T1)
                n185 = local read "Canal cero WS2"() -> (w381:bool)
                n186 = local read "Digital?"() -> (w394:bool)
                n187 = local read "RFID LR6 on?"() -> (w384:bool)
                n188 = xnode "Read/Write Control"("FPGA VI Reference In"=w409, "error in"=w408, "Data Rate"=w395, "Digital?"=w394, "Canal cero WS1?"=w393, "Count(mSec)"=w392, "Offset_WS1"=w382, "Offset_WS2"=w383, "Canal cero WS2?"=w381) -> ("FPGA VI Reference Out"=w399:refnum<k20>, "error out"=w398:errorcluster)
                n189 = case shown="False" w384 {
                  tunnel: [errorcluster {"status"=FALSE, "code"=0, "source"=""} ("error out") w414] -> w391
                  frame False {
                  }
                  frame True {
                    n190 = local read "RFID_LR6_Error"() -> (w415:errorcluster)
                    n191 = call "LH6HD.vi"("error in (no error)"=w415, "Action"=enum16{"Init", "Start", "Read", "Stop", "Exit"}."Start") -> ("error out"=w414:errorcluster)  [unwired: 8 in, 1 out]
                  }
                }
                n192 = Add(x="Nº inductivos", y="Nº de acelerómetros") -> (x+y=w386:i32)
                n193 = call "DMACalc.vi"("Number of Channels"=w386, "Number of Samples"=w388, "Rate (Hz)"=w400) -> ("Block Size"=w404:u32, "Time to Acquire Block (ms)"=w405:i32, "Host Buffer Size"=w410:u32)  [unwired: 6 in]
                n194 = call "Pathhorafech(SubVI)_varios.vi"("Folder path"=path "c:/Trenes", "Nº de acelerómetros"="Nº de acelerómetros", "Nº inductivos"="Nº inductivos") -> ("Acel_Paths"=w396:path[])  [unwired: 1 in, 1 out]
                "Nombre de archivo" <- w396
                n195 = for {
                  tunnel: w396 -> [w419] mode=indexing
                  tunnel: [w418] -> w403 mode=indexing
                  tunnel: [w417] -> w402
                  n196 = Open/Create/Replace File(file path (use dialog)=w419, operation (0:open)=T6."replace or create", access (0:read/write)=enum16{"read/write", "read-only", "write-only"}."read/write", disable buffering (F)=TRUE) -> (refnum out=w418:refnum<file>, error out=w417:errorcluster)  [unwired: 1 in, 2 out]
                }
                n197 = xnode "Invoke Method"("FPGA VI Reference In"=w399, "error in"=w398, "Requested Depth"=w410) -> ("FPGA VI Reference Out"=w412:refnum<k20>, "error out"=w411:errorcluster)  [unwired: 1 out]
                n198 = Get Date/Time In Seconds() -> (seconds since 1Jan1904=→"Inicio pasada":timestamp)
                n199 = xnode "Invoke Method"("FPGA VI Reference In"=w412, "error in"=w411) -> ("FPGA VI Reference Out"=w407:refnum<k20>, "error out"=w406:errorcluster)
              }
              frame #1 {
                n200 = while "Data Acquisition" {
                  tunnel: w438 -> [w493]
                  shift-right: [w518] -> _
                  shift-left: u32 0 ("t") -> [w514]
                  tunnel: w436 -> [w519]
                  tunnel: w435 -> [w517]
                  shift-right: [w520] -> w440
                  shift-left: w437 -> [w511]
                  tunnel: [w515] -> w441
                  tunnel: w434 -> [w497]
                  tunnel: [w498] -> w439
                  shift-right: [w496] -> w432
                  shift-left: w433 -> [w507]
                  i -> [w492]
                  stop <- w516 stop-if-true
                  # "Detector de presencia"
                  # "Mide el tiempo de paso del tren y con ello se puede calcular\nla velocidad la unidad"
                  n201 = xnode "Invoke Method"("FPGA VI Reference In"=w493, "error in"=w511, "Number of Elements"=w514, "Timeout (ms)"=0) -> ("FPGA VI Reference Out"=w489:refnum<k20>, "error out"=w495:errorcluster, "Data"=w510:fxp<+/-,24,4>[], "Elements Remaining"=w512:u32)
                  n202 = case "Data Ready" shown="Default" w514 {
                    tunnel: w519 -> [w542 _]
                    tunnel: [w541 u32 0 ("t")] -> w518
                    tunnel: w517 -> [w543 _]
                    tunnel: w512 -> [w540 _]
                    tunnel: w510 -> [_ w565]
                    tunnel: w507 -> [w539 w564]
                    tunnel: [w539 w566] -> w496
                    tunnel: w497 -> [w538 w563]
                    tunnel: [w538 w562] -> w498
                    frame 0 {
                      # "En este caso se compara los elementos que quedan\nen la FIFO del controlador con el tamaño dell bloque\nque aparece en el panel frontal. Si el número de \nelementos en la FIFO es mayor o igual que el tamaño\n del bloque se pasa al siguiente caso y se guardan \nlos datos en un archivo. El reloj que aparece es una\nespera para no consumir recursos."
                      n203 = Greater Or Equal?(x=w540, y=w543) -> (x >= y?=w544:bool)
                      n204 = case shown="False" w544 {
                        tunnel: [u32 0 ("Block Size") w548] -> w541
                        tunnel: [w547 0 ("t")] -> w545
                        tunnel: w542 -> [w547 _]
                        tunnel: w543 -> [_ w548]
                        frame False {
                        }
                        frame True {
                        }
                      }
                      n205 = call "WaitMinTimeBetweenCall.vi"("Minimum ms between calls"=w545) -> ()  [unwired: 2 in]
                    }
                    frame Default {
                      n206 = To Single Precision Float(number=w565) -> (single precision float=w552:sgl[])
                      n207 = Decimate 1D Array(w552) -> (w558:sgl[], w561:sgl[], w560:sgl[], w559:sgl[], w557:sgl[], w556:sgl[], w555:sgl[], w554:sgl[], w553:sgl[], w550:sgl[])
                      n208 = Build Array(w558, w561, w560, w559, w557, w556, w555, w554, w553, w550) -> (w551:sgl[][])
                      n209 = for {
                        tunnel: T7."little-endian" ("byte order (0:big-endian, network order)") -> [w575]
                        shift-right: [w569] -> w566
                        shift-left: w564 -> [w570]
                        tunnel: w551 -> [w573] mode=indexing
                        tunnel: w563 -> [w572] mode=indexing
                        tunnel: [w571] -> w562 mode=indexing
                        n210 = Write to Binary File(file (use dialog)=w572, data=w573, error in=w570, 5:FALSE ("prepend array or string size? (T)"), 9:w575) -> (refnum out=w571:refnum<file>, error out=w569:errorcluster)  [unwired: 2 out]
                      }
                    }
                  }
                  n211 = xnode "Read/Write Control"("FPGA VI Reference In"=w489, "error in"=w495) -> ("FPGA VI Reference Out"=w509:refnum<k20>, "error out"=w508:errorcluster, "Parar"=w485:bool, "Nº Ruedas 1"=→"Nº Ruedas 1":i32, "NºRuedas 2"=→"NºRuedas 2":i32)
                  "Parar" <- w485
                  n212 = case shown="False" w485 {
                    tunnel: [w524 w533] -> w486
                    tunnel: [w526 0.0] -> w501
                    frame False {
                      n213 = local read "Inicio pasada"() -> (w529:timestamp)
                      n214 = Get Date/Time In Seconds() -> (seconds since 1Jan1904=w528:timestamp)
                      n215 = To Double Precision Float(number=w528) -> (double precision float=w527:dbl)
                      n216 = To Double Precision Float(number=w529) -> (double precision float=w530:dbl)
                      n217 = Subtract(x=w527, y=w530) -> (x-y=w526:dbl)
                      "Tiempo de paso (s)" <- w526
                      n218 = local write "Tiempo"(w527) -> ()
                      n219 = local read "Boton Adquirir?"() -> (w521:bool)
                      n220 = Greater?(x=w526, y="Tiempo de adquisicion") -> (0:w523:bool)
                      n221 = Select(t=w523, s=w521, f=FALSE) -> (s? t:f=w524:bool)
                    }
                    frame True {
                      n222 = local read "Tiempo"() -> (w537:dbl)
                      n223 = local read "Tiempo extra al detector de paso (s)"() -> (w532:dbl)
                      n224 = Get Date/Time In Seconds() -> (seconds since 1Jan1904=w534:timestamp)
                      n225 = To Double Precision Float(number=w534) -> (double precision float=w535:dbl)
                      n226 = Subtract(x=w535, y=w537) -> (x-y=w536:dbl)
                      "Tiempo extra de adquisición (s)" <- w536
                      n227 = Greater?(x=w536, y=w532) -> (0:w533:bool)
                    }
                  }
                  "Fin" <- w486
                  n228 = local read "Timeout ruedas"() -> (w484:dbl)
                  n229 = xnode ("CheckLate")("FPGA VI Reference In"=w509, "error in"=w508) -> ("FPGA VI Reference Out"=w491:refnum<k20>, "error out"=w504:errorcluster, "Buffer Underflow"=→"Buffer Underflow":bool, "Buffer Overflow"=w494:bool)
                  "Buffer Overflow" <- w494
                  n230 = Greater?(x=w501, y=w484) -> (0:w499:bool)
                  "Timeout ruedas" <- w499
                  n231 = call "ErrorOverFlow.vi"("Buffer Overflow"=w494) -> ("error out"=w502:errorcluster)
                  n232 = call "ErrorUnderFlow.vi"() -> ("error out"=w503:errorcluster)  [unwired: 1 in]
                  n233 = Merge Errors(w504, w503, w502) -> (w490:errorcluster)
                  n234 = Unbundle By Name(w496) -> ("status"=w500:bool)
                  n235 = Unbundle By Name(w490) -> ("status"=w506:bool)
                  n236 = Compound Arithmetic op=OR(w506, w486, w499, w500) -> (w516:bool)
                  "result" <- w516
                  n237 = case "Flush" shown="True" w516 {
                    tunnel: [w576 w581] -> w520
                    tunnel: [w577 w580] -> w515
                    tunnel: w491 -> [w577 w579]
                    tunnel: w490 -> [w576 w578]
                    frame False {
                    }
                    frame True {
                      n238 = xnode "Invoke Method"("FPGA VI Reference In"=w579, "error in"=w578) -> ("FPGA VI Reference Out"=w580:refnum<k20>, "error out"=w581:errorcluster)
                    }
                  }
                  "Block Size" <- w517
                  "Time to Acquire Block (ms)" <- w519
                  "Numeric 3" <- w492
                }
                n239 = call <vilib>:"Watchdog Whack.vi"("error in (no error)"=w427, "reset watchdog after expire? (F)"=TRUE, "watchdogID in"=w428) -> ("error out"=w424:errorcluster, "watchdogID out"=w425:u64)  [unwired: 2 in, 1 out]
                n240 = local read "RFID LR6 on?"() -> (w423:bool)
                n241 = case shown="True" w423 {
                  tunnel: w430 -> [w442 w448]
                  tunnel: [w442 w447] -> w429
                  frame False {
                  }
                  frame True {
                    n242 = while {
                      shift-right: [w455] -> w447
                      shift-left: w448 -> [w456]
                      shift-right: [w454] -> w445
                      shift-left: string[] [] -> [w453]
                      shift-right: [w449] -> w443
                      shift-left: i32[] [] -> [w450]
                      i -> [w451]
                      stop <- w452 stop-if-true
                      n243 = case shown="No Error" w456 {
                        selector: w456 -> [w467 _]
                        tunnel: [w466 w482] -> w455
                        tunnel: [w462 string[] []] -> w454
                        tunnel: w453 -> [w461 _]
                        tunnel: w451 -> [w460 _]
                        tunnel: w450 -> [w459 _]
                        tunnel: [w458 i32[] []] -> w449
                        frame No Error {
                          n244 = call "LH6HD.vi"("error in (no error)"=w467, "Action"=enum16{"Init", "Start", "Read", "Stop", "Exit"}."Read") -> ("error out"=w466:errorcluster, "Tag"=w463:string)  [unwired: 8 in]
                          n245 = Not Equal?(x="", y=w463) -> (x != y?=w464:bool)
                          n246 = case shown="False" w464 {
                            tunnel: w463 -> [_ w476]
                            tunnel: [w470 w475] -> w462
                            tunnel: w461 -> [w470 w474]
                            tunnel: w460 -> [_ w471]
                            tunnel: w459 -> [w469 w473]
                            tunnel: [w469 w472] -> w458
                            frame False {
                            }
                            frame True {
                              n247 = Build Array (concatenate)(w474, w476) -> (w475:string[])
                              n248 = Build Array (concatenate)(w473, w471) -> (w472:i32[])
                            }
                          }
                        }
                        frame Error {
                          n249 = local read "LR6 IP address"() -> (w479:string)
                          n250 = local read "DeviceAddress"() -> (w477:u8)
                          n251 = local read "Port LR6"() -> (w480:u16)
                          n252 = call "LH6HD.vi"("DeviceAddress"=w477, "Reader Port"=w480, "IP Address"=w479, "Action"=enum16{"Init", "Start", "Read", "Stop", "Exit"}."Init") -> ("error out"=w482:errorcluster)  [unwired: 6 in, 1 out]
                        }
                      }
                      n253 = Wait Until Next ms Multiple(millisecond multiple=u32 500) -> ()  [unwired: 1 out]
                      n254 = local read "result"() -> (w452:bool)
                      "it-LR6" <- w451
                    }
                    "TAGs LR6" <- w445
                    "it-read-LR6" <- w443
                  }
                }
              }
              frame #2 {
                n255 = local read "RFID LR6 on?"() -> (w585:bool)
                n256 = Array Size(array=w605) -> (size(s)=w603:i32)
                n257 = local read "TAGs LR6"() -> (w592:string[])
                n258 = local read "timeout ms (60000)"() -> (w588:i32)
                n259 = local read "bytes to read"() -> (w587:i32)
                n260 = local read "RFID NEM on?"() -> (w586:bool)
                n261 = Decrement(x=w603) -> (x-1=w604:i32)
                n262 = local read "Puerto RFID"() -> (w620:u16)
                n263 = case shown="False" w585 {
                  tunnel: w599 -> [w645 w647]
                  tunnel: [w645 w646] -> w598
                  frame False {
                  }
                  frame True {
                    n264 = call "LH6HD.vi"("error in (no error)"=w647, "Action"=enum16{"Init", "Start", "Read", "Stop", "Exit"}."Stop") -> ("error out"=w646:errorcluster)  [unwired: 8 in, 1 out]
                  }
                }
                n265 = local read "RFID_Error"() -> (w631:errorcluster)
                n266 = local read "IP RFID"() -> (w602:string)
                n267 = local read "RFID_ID"() -> (w630:refnum<k5>)
                n268 = Index Array(array=w605, index=w604) -> (element=w613:refnum<file>)
                n269 = local write "result"(FALSE ("result")) -> ()
                n270 = case shown="True" w586 {
                  tunnel: [_ w660] -> w632
                  tunnel: w631 -> [w650 w659]
                  tunnel: w630 -> [w649 w658]
                  tunnel: [w649 w657] -> w629
                  tunnel: [w650 w656] -> w624
                  tunnel: w620 -> [_ w655]
                  tunnel: w602 -> [_ w654]
                  tunnel: [_ w653] -> w582
                  tunnel: w588 -> [_ w652]
                  tunnel: w587 -> [_ w651]
                  frame False {
                  }
                  frame True {
                    n271 = call "RFID_28_03_12.vi"("BYTES TO READ"=w651, "TIMEOUT"=w652, "RFID_Error"=w659, "Puerto RFID"=w655, "IP RFID"=w654, "RFID ID"=w658) -> ("RFID Error"=w656:errorcluster, "connection ID out"=w657:refnum<k5>, "TAGs HEX"=w653:string[], "Unidad"=w660:u32)  [unwired: 1 in]
                  }
                }
                "TAGs HEX" <- w582
                n272 = local write "RFID_LR6_Error"(w598) -> ()
                n273 = for {
                  tunnel: w592 -> [w663] mode=indexing
                  tunnel: [w661] -> w591 mode=indexing
                  n274 = Search and Replace String(input string=w663, search string="00") -> (result string=w661:string)  [unwired: 6 in, 3 out]
                }
                n275 = xnode "Read/Write Control"("FPGA VI Reference In"=w584, "error in"=w583) -> ("FPGA VI Reference Out"=w634:refnum<k20>, "error out"=w633:errorcluster, "Chassis Temperature"=w643:i16)
                n276 = Index Array(array=w582) -> (element=w597:string)  [unwired: 1 in]
                n277 = Not Equal?(x=w597, y="" ("delimiter (\\t)")) -> (x != y?=w595:bool)
                "Plataformas?" <- w595
                n278 = case shown="True" w595 {
                  tunnel: w591 -> [w664 w665]
                  tunnel: [w664 w667] -> w600
                  tunnel: w582 -> [_ w666]
                  frame False {
                  }
                  frame True {
                    n279 = call "Union_TAGs_RFIDs.vi"("TAGs LR6"=w665, "TAGs HEX"=w666) -> ("TAGs"=w667:string[])
                  }
                }
                "TAGs" <- w600
                n280 = Divide(x=w643, y=4.0) -> (x/y=w644:dbl)
                "Temperatura (ºC)" <- w644
                n281 = local read "Tiempo de paso (s)"() -> (w627:dbl)
                n282 = local read "Nombre de archivo"() -> (w612:path[])
                n283 = Multiply(x=w627, y=1000.0) -> (x*y=w625:dbl)
                n284 = for {
                  shift-right: [w673] -> w618
                  shift-left: string[] [] -> [w672]
                  tunnel: w600 -> [w671] mode=indexing
                  n285 = Insert Into Array(array=w672, new element=w671) -> (w673:string[])  [unwired: 1 in]
                }
                n286 = Build Array(w644, w625, w632) -> (w638:dbl[])
                n287 = local write "RFID_ID"(w629) -> ()
                n288 = local write "RFID_Error"(w624) -> ()
                n289 = Delete From Array(array=w612) -> (deleted portion=w611:path)  [unwired: 2 in, 1 out]
                n290 = To Single Precision Float(number=w638) -> (single precision float=w641:sgl[])
                n291 = xnode "Read/Write Control"("FPGA VI Reference In"=w634, "error in"=w633, "Stop"=TRUE ("stop")) -> ("FPGA VI Reference Out"=w615:refnum<k20>, "error out"=w614:errorcluster)
                n292 = Path To String(path=w611) -> (string=w617:string)
                n293 = Write to Binary File(file (use dialog)=w613, data=w641, error in=w637, 5:FALSE ("prepend array or string size? (T)"), 9:T7."little-endian" ("byte order (0:big-endian, network order)")) -> (error out=w610:errorcluster)  [unwired: 3 out]
                n294 = local read "Timeout ruedas"() -> (w628:bool)
                n295 = Build Array (concatenate)(w617, w618) -> (w593:string[])
                n296 = local read "TAGS leidos"() -> (w606:path)
                n297 = for {
                  shift-right: [w670] -> w621
                  shift-left: w610 -> [w669]
                  tunnel: w605 -> [w668] mode=indexing
                  n298 = Close File(refnum=w668, error in=w669) -> (error out=w670:errorcluster)  [unwired: 1 out]
                }
                n299 = xnode "Invoke Method"("FPGA VI Reference In"=w615, "error in"=w614) -> ("FPGA VI Reference Out"=w623:refnum<k20>, "error out"=w622:errorcluster)
                n300 = call-poly <vilib>:"Write Delimited Spreadsheet.vi"("file path (dialog if empty)"=w606, "1D data"=w593, "append to file? (F)"=TRUE ("transpose? (no:F)"), "transpose? (F)"=TRUE ("append to file? (new file:F)"), "delimiter (\\t)"=";" ("delimiter (\\t)")) -> ()  [unwired: 9 in, 2 out]
                n301 = Select(t="TEST", s=w628, f="Procesado") -> (s? t:f=w635:string)
              }
            }
            n302 = call <vilib>:"Watchdog Clear.vi"("error in (no error)"=w346, "watchdogID in"=w347) -> ("error out"=w348:errorcluster)  [unwired: 5 in]
            n303 = Unbundle By Name(w373) -> ("status"=w362:bool)
            n304 = Unbundle By Name(w371) -> ("status"=w363:bool)
            n305 = Merge Errors(w371, w348) -> (w370:errorcluster)
            n306 = Compound Arithmetic op=OR(w362, w363) -> (w360:bool)
            n307 = Select(t="TEST", s=w360, f=w361) -> (s? t:f=w358:string)
          }
          frame "Procesado" {
            n308 = local read "Watchdog config"() -> (w680:T3)
            n309 = call <vilib>:"Watchdog Configure.vi"("error in (no error)"=w683, "expiration actions"=w680, "timeout (1 sec)"=300.0) -> ("error out"=w682:errorcluster, "watchdogID"=w679:u64)  [unwired: 1 in, 2 out]
            n310 = flat-sequence {
              tunnel: w682 -> [w705]
              tunnel: [w708] -> w685
              tunnel: w679 -> [w700]
              tunnel: [w699] -> w678
              tunnel: [w698] -> w677
              tunnel: [w913] -> w695
              tunnel: w685 -> [w913]
              tunnel: [w907] -> w676
              tunnel: w678 -> [w907]
              tunnel: [w906] -> w675
              tunnel: w677 -> [w906]
              frame #0 {
                n311 = flat-sequence {
                  tunnel: [w779] -> w707
                  tunnel: [w764] -> w706
                  tunnel: w705 -> [w729]
                  tunnel: [w767] -> w704
                  tunnel: [w754] -> w701
                  tunnel: [w766] -> w703
                  tunnel: [w753] -> w702
                  tunnel: w700 -> [w730]
                  tunnel: [w727] -> w699
                  tunnel: [w726] -> w698
                  frame #0 {
                    # "No es necesario leer el segundo archivo"
                    # "Distancia de\nla unidad"
                    n312 = local read "Nombre de archivo"() -> (w720:path[])
                    n313 = local read "Tabla_flota"() -> (w763:string[][])
                    n314 = call <vilib>:"Watchdog Whack.vi"("error in (no error)"=w729, "reset watchdog after expire? (F)"=TRUE, "watchdogID in"=w730) -> ("error out"=w726:errorcluster, "watchdogID out"=w727:u64)  [unwired: 2 in, 1 out]
                    n315 = local read "TAGs"() -> (w757:string[])
                    n316 = call "Series_ejes_flota.vi"("Tabla_flota"=w763, "Tags"=w757) -> ("Nº Ejes"=w719:i32[], "Series del convoy"=w756:string[])  [unwired: 2 in, 1 out]
                    "Nº Ejes" <- w719
                    n317 = local read "Puntos medios de las ventanas"() -> (w765:dbl[][])
                    n318 = Array Size(array=w720) -> (size(s)=w773:i32)
                    n319 = Add Array Elements(numeric array=w719) -> (sum=w725:i32)
                    "Ejes_convoy" <- w725
                    n320 = Subtract(x=w773, y=2 ("length")) -> (x-y=w775:i32)
                    n321 = Array Size(array=w756) -> (size(s)=→"Nº UTs":i32)
                    n322 = Delete From Array(array=w720, length=2, index=w775) -> (deleted portion=w743:path[], array with subset deleted=w766:path[])
                    n323 = Index Array(array=w743) -> (element #1=w721:path, element #2=w722:path)  [unwired: 2 in]
                    n324 = local read "Frecuencia de muestreo (Hz)"() -> (w710:dbl)
                    n325 = Read from Binary File(5:sgl 0.0, 9:T7."little-endian" ("byte order (0:big-endian, network order)"), 10:-1 ("count (1)"), 11:w722) -> (0:w771:errorcluster, 2:w745:sgl[], 3:w772:refnum<file>)  [unwired: 1 in, 2 out]
                    n326 = local read "Series_flota"() -> (w762:string[])
                    n327 = local read "Offset_rueda WS 2"() -> (w711:fxp<+/-,24,-4>)
                    n328 = Close File(refnum=w772, error in=w771) -> (error out=w767:errorcluster)  [unwired: 1 out]
                    n329 = Read from Binary File(5:sgl 0.0, 9:T7."little-endian" ("byte order (0:big-endian, network order)"), 10:-1 ("count (1)"), 11:w721) -> (0:w741:errorcluster, 2:w733:sgl[], 3:w742:refnum<file>)  [unwired: 1 in, 2 out]
                    n330 = Array Size(array=w745) -> (size(s)=w761:i32)
                    n331 = Close File(refnum=w742, error in=w741) -> ()  [unwired: 2 out]
                    n332 = Subtract(x=w761, y=3 ("length")) -> (x-y=w759:i32)
                    n333 = Array Size(array=w733) -> (size(s)=w737:i32)
                    n334 = Delete From Array(array=w745, length=3, index=w759) -> (deleted portion=→"deleted portion":sgl[], array with subset deleted=w717:sgl[])
                    n335 = call "Distancias_ejes_convoy.vi"("Series_flota1"=w756, "Ejes_UT"=w719, "Puntos medios de las ventanas"=w765, "Series_flota"=w762) -> ("Distancias_entre_ejes_convoy"=w764:dbl[])  [unwired: 1 in]
                    n336 = Subtract(x=w737, y=3 ("length")) -> (x-y=w735:i32)
                    n337 = Delete From Array(array=w733, length=3, index=w735) -> (deleted portion=→"deleted portion 2":sgl[], array with subset deleted=w732:sgl[])
                    n338 = call "Analogico_digital.vi"("Array"=w717, "Offset WS"=w711, "Frecuencia muestreo"=w710) -> ("array w/ subset deleted"=w712:sgl[], "Tiempo\npaso"=w709:dbl)  [unwired: 6 in]
                    "Waveform Graph 2" <- w712
                    n339 = call "Puntos medio de pulso.vi"("DI Inductivo"=w712) -> ("Puntos"=w779:sgl[], "Número de ejes"=w746:i32)  [unwired: 1 in]
                    "Número de ejes detectados" <- w746
                    n340 = Build Array(w717, w732) -> (→"Waveform Graph":sgl[][])
                    n341 = local read "TAGs"() -> (w752:string[])
                    n342 = local read "it-LR6"() -> (w749:i32)
                    n343 = local read "it-read-LR6"() -> (w750:i32[])
                    n344 = local read "TAGs LR6"() -> (w751:string[])
                    n345 = local read "Plataformas?"() -> (w748:bool)
                    n346 = Decrement(x=w746) -> (x-1=w778:i32)
                    n347 = disable-structure shown="Enabled" {
                      disable-tunnel: w717 -> [w788 w791]
                      disable-tunnel: [FALSE ("element") TRUE ("element")] -> w714
                      disable-tunnel: [w782 w790] -> w713
                      frame Disabled {
                        n348 = Equal?(x=w788, y=0.0) -> (x = y?=w785:bool[])
                        n349 = Equal?(x=w788, y=1.0) -> (x = y?=w786:bool[])
                        n350 = Or(x=w785, y=w786) -> (x .or. y?=w782:bool[])
                      }
                      frame Enabled {
                        n351 = Greater?(x=w791, y=0.1) -> (0:w790:bool[])
                      }
                    }
                    n352 = call "Calculo_Velocidad.vi"("Tiempo de paso (s)"=w709, "Ejes"=w778, "Puntos iniciales de las ventanas"=w764) -> ("V (m/s)"=→"V (m/s)":dbl, "Longitud de la unidad"=→"Longitud de la unidad":dbl)
                    n353 = call "TAGs_AURAwheel.vi"("Nº Ejes"=w719, "TAGs"=w752, "Ejes_convoy"=w725, "it-LR6"=w749, "TAGs LR6"=w751, "it-read-LR6"=w750, "Plataformas?"=w748) -> ("TAGS_AURA"=→"TAGs_AURAwheel":string[][])  [unwired: 1 in]
                    n354 = Get Volume Info(11:path "c:/" ("path")) -> (1:→"Disco Duro Disponible (bytes)":i64)  [unwired: 1 in, 5 out]
                    n355 = Equal?(x=w725, y=w746) -> (x = y?=w753:bool)
                    n356 = Search 1D Array(1D array=w713, element=w714) -> (index of element=w715:i32)  [unwired: 1 in]
                    n357 = Equal?(x=w715, y=-1) -> (x = y?=w718:bool)
                    n358 = And(x=w753, y=w718) -> (x .and. y?=w754:bool)
                    "Archivo\nvalido?" <- w754
                  }
                }
                n359 = case shown="True" w701 {
                  tunnel: w704 -> [w795 w826]
                  tunnel: [w795 w825] -> w708
                  tunnel: w707 -> [_ w830]
                  tunnel: w706 -> [_ w828]
                  tunnel: w703 -> [_ w829]
                  tunnel: w702 -> [w793 _]
                  frame False {
                    n360 = local read "Nombre de archivo"() -> (w794:path[])
                    n361 = for {
                      tunnel: w794 -> [w797] mode=indexing
                      tunnel: w793 -> [w796]
                      n362 = flat-sequence {
                        tunnel: w797 -> [w807]
                        tunnel: [w807] -> w800
                        tunnel: [w806] -> w799
                        tunnel: w796 -> [w805]
                        tunnel: w800 -> [w814]
                        tunnel: [w813] -> w798
                        tunnel: w799 -> [w813]
                        tunnel: w798 -> [w816]
                        frame #0 {
                          w806 = path "c:/Est_Adq.csv" ("file path (use dialog)")
                          n363 = Path To String(path=w807) -> (string=w808:string)
                          n364 = Select(t="Nº Ejes detectados WS diferente a Nº Ejes TAGs" ("delimiter (\\t)"), s=w805, f="La señal del inductivo no es digital" ("delimiter (\\t)")) -> (s? t:f=w802:string)
                          n365 = Build Array(w808, w802) -> (w801:string[])
                          n366 = call-poly <vilib>:"Write Delimited Spreadsheet.vi"("file path (dialog if empty)"=w806, "1D data"=w801, "append to file? (F)"=FALSE ("transpose? (no:F)"), "transpose? (F)"=TRUE ("append to file? (new file:F)"), "delimiter (\\t)"=";" ("delimiter (\\t)")) -> ()  [unwired: 9 in, 2 out]
                        }
                        frame #1 {
                          n367 = local read "Borrar archivos\nadquisicion con error"() -> (w812:bool)
                          n368 = case shown="True" w812 {
                            tunnel: w814 -> [_ w815]
                            frame False {
                            }
                            frame True {
                              n369 = Delete(path (use dialog)=w815) -> ()  [unwired: 1 in, 6 out]
                            }
                          }
                        }
                        frame #2 {
                          n370 = File/Directory Info(path=w816) -> (size=w819:i64)  [unwired: 1 in, 6 out]
                          n371 = Greater?(x=w819, y=i64 1000000) -> (0:w817:bool)
                          n372 = case shown="True" w817 {
                            tunnel: w816 -> [_ w820]
                            frame False {
                            }
                            frame True {
                              n373 = Delete(path (use dialog)=w820) -> ()  [unwired: 4 in, 3 out]
                            }
                          }
                        }
                      }
                    }
                  }
                  frame True {
                    n374 = flat-sequence {
                      tunnel: w830 -> [w900]
                      tunnel: w829 -> [w897]
                      tunnel: w828 -> [w901]
                      tunnel: [w885] -> w827
                      frame #0 {
                        # "SALIDA \n\nMáximos por rueda inductivo"
                        # "8 acelerómetros"
                        # "Velocidad"
                        n375 = local read "Frecuencia de muestreo (Hz)"() -> (w899:dbl)
                        n376 = local read "Distancia de acelerómetros"() -> (w889:dbl[])
                        n377 = local read "Parámetros acelerómetros"() -> (w896:dbl[])
                        n378 = local read "Número de ejes detectados"() -> (w895:i32)
                        n379 = local read "Distancias generales"() -> (w894:dbl[])
                        n380 = local read "dt RMS"() -> (w898:dbl)
                        n381 = local read "Direccion 0?"() -> (w886:bool)
                        n382 = Index Array(array=w894, index=1) -> (element=w892:dbl)
                        n383 = Select(t=0.0, s=w886, f=w892) -> (s? t:f=w890:dbl)
                        n384 = Subtract(x=w890, y=w889) -> (x-y=w888:dbl[])
                        n385 = Absolute Value(x=w888) -> (abs(x)=w887:dbl[])
                        n386 = call "Procesado_aRMS_BIdirecc.vi"("Paths_canales_aRMS"=w897, "Ejes Procesados"=w895, "Distancias\nacelerometros"=w887, "Distancias generales (m)"=w894, "Distancias centrales de las ruedas\n               configuración (m)"=w901, "Frecuencia de muestreo"=w899, "Parámetros acelerómetros"=w896, "dt RMS 2"=w898, "Puntos"=w900) -> ("Max RMS Ruedas"=w884:dbl[][])  [unwired: 2 in]
                        n387 = Transpose 2D Array(2D array=w884) -> (transposed array=w885:dbl[][])
                        "Max RMS Ruedas" <- w885
                      }
                    }
                    n388 = local read "Use Aura?"() -> (w824:bool)
                    n389 = local read "TAGs_AURAwheel"() -> (w822:string[][])
                    n390 = local read "Nº Ejes"() -> (w821:i32[])
                    n391 = for {
                      tunnel: w824 -> [w835]
                      tunnel: [w834] -> w823 mode=indexing
                      tunnel: w822 -> [w833] mode=indexing
                      shift-right: [w832] -> _
                      shift-left: w827 -> [w836]
                      tunnel: w821 -> [w831] mode=indexing
                      # "dev.api.aurawheel.com"
                      n392 = case shown="True" w835 {
                        tunnel: w836 -> [w837 w849]
                        tunnel: [errorcluster {"status"=FALSE, "code"=0, "source"=""} ("error out") w854] -> w834
                        tunnel: w833 -> [_ w850]
                        tunnel: [w837 w848] -> w832
                        tunnel: w831 -> [_ w846]
                        frame False {
                        }
                        frame True {
                          w858 = cluster{"status":string} {"status"=""}
                          n393 = local read "Parametros AuraWheel"() -> (w883:string[])
                          n394 = Delete From Array(array=w849, length=w846, index (row)=0) -> (deleted portion=w845:dbl[][], array with subset deleted=w848:dbl[][])  [unwired: 1 in]
                          n395 = Get Date/Time In Seconds() -> (seconds since 1Jan1904=w879:timestamp)
                          n396 = Format Date/Time String(time format string (%c)="%H:%M:%S%3u", seconds (now)=w879) -> (date/time string=w877:string)  [unwired: 1 in]
                          n397 = Get Date/Time In Seconds() -> (seconds since 1Jan1904=w853:timestamp)
                          n398 = Scan From String(format string="%d:%d:%f", input string=w877) -> (output 1=w874:i32, output 2=w873:i32, output 3=w871:dbl)  [unwired: 5 in, 3 out]
                          n399 = local read "V (m/s)"() -> (w841:dbl)
                          n400 = local read "Temperatura (ºC)"() -> (w851:dbl)
                          n401 = Multiply(x=w841, y=3.6) -> (x*y=w839:dbl)
                          n402 = Multiply(x=w871, y=1000.0) -> (x*y=w867:dbl)
                          n403 = call "Time_to_ms.vi"("seconds since 1Jan1904"=w853) -> ("Numeric"=w852:dbl)  [unwired: 1 in]
                          n404 = Multiply(x=w873, y=60000) -> (x*y=w868:i32)
                          n405 = Multiply(x=3600000, y=w874) -> (x*y=w869:i32)
                          n406 = Index Array(array=w883) -> (element #1=w844:string, element #2=w843:string, element #3=w842:string)  [unwired: 3 in]
                          n407 = call "aw_WRDCluster_8acel.vi"("Array TAGs"=w850, "Max RMS Ruedas"=w845, "TimeStamp"=w852, "p_sp"=w839, "p_tp"=w851) -> ("JSON cluster"=w880:T9)  [unwired: 1 in]
                          n408 = Compound Arithmetic op=ADD(w869, w868, w867) -> (w866:dbl)
                          n409 = To Variant(anything=w880) -> (Variant=w863:variant)
                          n410 = To Unsigned Long Integer(number=w866) -> (unsigned 32bit integer=w865:u32)
                          n411 = call "gjson_Create.vi"("JSON Object in"=w863) -> ("error out"=w861:errorcluster, "JSON String Out"=w862:string)  [unwired: 9 in]
                          n412 = Number To Decimal String(number=w865) -> (decimal integer string=w864:string)  [unwired: 1 in]
                          n413 = To Variant(anything=w858) -> (Variant=w857:variant)
                          n414 = call "aw_SendData.vi"("pwd"=w844, "x-nem-datetime"=w864, "User"=w843, "error in"=w861, "JSON Object"=w862, "URL"=w842) -> ("error out"=w859:errorcluster, "Response JSON"=w860:string, "Response headers"=→"Response headers":string)  [unwired: 3 in]
                          n415 = call "gjson_Parse.vi"("error in"=w859, "JSON String In"=w860, "JSON Cluster"=w857) -> ("error out"=w855:errorcluster, "JSON Cluster Out"=w856:variant)  [unwired: 7 in]
                          n416 = Variant To Data(error in=w855, type=w858, Variant=w856) -> (data=→"data":cluster{"status":string}, error out=w854:errorcluster)
                          "error AURA" <- w854
                        }
                      }
                    }
                    n417 = Merge Errors(w823, w826) -> (w825:errorcluster)
                  }
                }
              }
              frame #1 {
                n418 = local read "Bytes libre despues de borrar"() -> (w903:u32)
                n419 = local read "Archivo\nvalido?"() -> (w902:bool)
                n420 = local read "Bytes min libre"() -> (w904:u32)
                n421 = local read "Max archivos"() -> (w905:u32)
                n422 = local read "TAGS leidos"() -> (w909:path)
                n423 = File/Directory Info(path=w909) -> (size=w912:i64)  [unwired: 1 in, 6 out]
                n424 = local read "Path TEST"() -> (w908:path)
                n425 = case shown="True" w902 {
                  frame False {
                  }
                  frame True {
                    n426 = local read "Nombre de archivo"() -> (w915:path[])
                    n427 = call "Comprimir_a_1_archivo.vi"("Acel_paths"=w915) -> ("path_Pasada"=→"created path":path)
                  }
                }
                n428 = Greater?(x=w912, y=i64 1000000) -> (0:w910:bool)
                n429 = case shown="True" w910 {
                  tunnel: w909 -> [_ w916]
                  frame False {
                  }
                  frame True {
                    n430 = Delete(path (use dialog)=w916) -> ()  [unwired: 4 in, 3 out]
                  }
                }
                n431 = call "BORRADO_MEJORADO_Gonzalo.vi"("Bytes LIBRE OK"=w903, "Bytes Minimo de Memoria libre"=w904) -> ()  [unwired: 10 in]
                n432 = call "Borrar_carpeta.vi"("Nº Archivos Max"=w905, "Path Carpeta"=w908) -> ()  [unwired: 1 in]
              }
            }
            n433 = call <vilib>:"Watchdog Clear.vi"("error in (no error)"=w675, "watchdogID in"=w676) -> ("error out"=w674:errorcluster)  [unwired: 5 in]
            n434 = local read "RFID_Error"() -> (w686:errorcluster)
            n435 = Merge Errors(w695, w674) -> (w687:errorcluster)
            n436 = Merge Errors(w684, w686, w687) -> (w696:errorcluster)
            n437 = Unbundle By Name(w696) -> ("status"=w690:bool)
            n438 = Select(t="Descarga datos", s=FALSE, f="Espera") -> (s? t:f=w692:string)
            n439 = Select(t="TEST", s=w690, f=w692) -> (s? t:f=w689:string)
          }
          frame "TEST" {
            n440 = local read "Watchdog config"() -> (w925:T3)
            n441 = call <vilib>:"Watchdog Configure.vi"("expiration actions"=w925, "timeout (1 sec)"=200.0) -> ("error out"=w926:errorcluster, "watchdogID"=w923:u64)  [unwired: 2 in, 2 out]
            n442 = flat-sequence {
              tunnel: [w941] -> w930
              tunnel: w926 -> [w936]
              tunnel: w928 -> [w955]
              tunnel: [w954] -> w918
              tunnel: [w937] -> w927
              tunnel: w923 -> [w935]
              tunnel: [w934] -> w921
              tunnel: w922 -> [w933]
              tunnel: [w932] -> w920
              frame #0 {
                n443 = call <vilib>:"Watchdog Whack.vi"("error in (no error)"=w936, "reset watchdog after expire? (F)"=TRUE, "watchdogID in"=w935) -> ("error out"=w932:errorcluster, "watchdogID out"=w934:u64)  [unwired: 2 in, 1 out]
                n444 = Get Date/Time In Seconds() -> (seconds since 1Jan1904=w948:timestamp)
                n445 = local read "Ultimo TEST"() -> (w949:timestamp)
                n446 = To Double Precision Float(number=w948) -> (double precision float=w950:dbl)
                n447 = Subtract(x=w950, y=3600.0) -> (x-y=w952:dbl)
                n448 = To Time Stamp(1:w952) -> (0:w953:timestamp)
                n449 = In Range and Coerce(upper limit=w948, x=w949, lower limit=w953) -> (In Range?=w947:bool)  [unwired: 1 out]
                n450 = case shown="False" w947 {
                  tunnel: w933 -> [w984 _]
                  tunnel: w955 -> [w960 w999]
                  tunnel: [w969 errorcluster {"status"=FALSE, "code"=0, "source"=""} ("error out")] -> w954
                  tunnel: [w960 w999] -> w937
                  frame False {
                    n451 = local read "Timeout ruedas"() -> (w961:bool)
                    n452 = local read "Aviso no detección"() -> (w967:string)
                    n453 = local read "Aviso temperatura"() -> (w966:string)
                    n454 = case shown="True" w961 {
                      selector: w961 -> [_ w996]
                      tunnel: ["\r" w997] -> w959
                      frame False {
                      }
                      frame True {
                        w986 = "\n"
                        n455 = local read "Nº Ruedas 1"() -> (w993:i32)
                        n456 = local read "NºRuedas 2"() -> (w988:i32)
                        n457 = call "ErrorRuedas.vi"("Buffer Overflow"=w996) -> ("error out"=w998:errorcluster)
                        n458 = Number To Decimal String(number=w993) -> (decimal integer string=w991:string)  [unwired: 1 in]
                        n459 = Number To Decimal String(number=w988) -> (decimal integer string=w987:string)  [unwired: 1 in]
                        n460 = Concatenate Strings("Error Wheel sensors", "\n", "WS1 (ruedas):", w991, w986, "WS2 (ruedas):", w987, w986) -> (w989:string)
                        n461 = call "Error.vi"("Error con..."=w989, "error comunicacion 2"=w998) -> ("String"=w997:string)
                      }
                    }
                    n462 = local read "RFID_Error"() -> (w963:errorcluster)
                    n463 = local read "RFID_LR6_Error"() -> (w957:errorcluster)
                    n464 = local read "DC OK"() -> (w965:string)
                    n465 = call "Cabecera.vi"() -> ("String"=w982:string)
                    n466 = call "Adquisicion.vi"("Aviso no detección"=w967) -> ("String"=w981:string)
                    n467 = call "Temperatura.vi"("Aviso temperatura"=w966) -> ("String"=w980:string)
                    n468 = call "Fuente.vi"("DC OK"=w965) -> ("String"=w979:string)
                    n469 = call "FPGA.vi"("error out"=w960) -> ("String"=w978:string)
                    n470 = call "Escritura.vi"("error out"=w984) -> ("String"=w977:string)
                    n471 = call "Error.vi"("Error con..."="Error con el lecto RFID NEM", "error comunicacion 2"=w963) -> ("String"=w962:string)
                    n472 = call "Error.vi"("Error con..."="Error con el lecto RFID LR6-HD", "error comunicacion 2"=w957) -> ("String"=w956:string)
                    n473 = Concatenate Strings(w982, w981, w980, w979, w978, w977, w962, w956, w959) -> (w983:string)
                    n474 = call "STRINGhorafechA(SubVI).vi"() -> ("STRINGhora_fecha"=w976:string)
                    n475 = Concatenate Strings(w976, ".txt" ("string")) -> (w972:string)
                    n476 = Get Date/Time In Seconds() -> (seconds since 1Jan1904=→"Ultimo TEST":timestamp)
                    n477 = Build Array("c", "TEST" ("element"), w972) -> (w974:string[])
                    n478 = Array of Strings to Path(0:w974) -> (2:w970:path)  [unwired: 1 out]
                    n479 = Write to Text File(file (use dialog)=w970, text=w983) -> (error out=w969:errorcluster)  [unwired: 1 in, 3 out]
                  }
                  frame True {
                  }
                }
                n480 = local read "Fallo fotocelula"() -> (w940:bool)
                n481 = Unbundle By Name(w937) -> ("status"=w938:bool)
                n482 = local read "T fuera rango"() -> (w946:bool)
                n483 = Compound Arithmetic op=OR(w938, w940) -> (w939:bool)
                n484 = local write "Reset del controlador"(w939) -> ()
                n485 = Select(t="Escape", s=w946, f="Espera") -> (s? t:f=w943:string)
                n486 = Select(t="Configuracion", s=w939, f=w943) -> (s? t:f=w941:string)
              }
            }
            n487 = call <vilib>:"Watchdog Clear.vi"("error in (no error)"=w920, "watchdogID in"=w921) -> ("error out"=w919:errorcluster)  [unwired: 5 in]
            n488 = Merge Errors(w919, w918) -> (w917:errorcluster)
          }
          frame "Calibracion" {
            n489 = while {
              shift-right: [w1007] -> _
              shift-left: w1002 -> [w1005]
              shift-right: [w1012] -> _
              shift-left: w1001 -> [w1004]
              stop <- "stop" stop-if-true
              n490 = xnode "Invoke Method"("FPGA VI Reference In"=w1005, "error in"=w1004) -> ("FPGA VI Reference Out"=w1006:refnum<k20>, "error out"=w1003:errorcluster)  [unwired: 1 in]
              n491 = xnode "Read/Write Control"("FPGA VI Reference In"=w1006, "error in"=w1003) -> ("FPGA VI Reference Out"=w1010:refnum<k20>, "error out"=w1009:errorcluster, "Chassis Temperature"=→"Chassis \nTemperature":i16)
              "error out" <- w1009
              n492 = case shown="True" "Adquirir 2" {
                tunnel: w1010 -> [w1016 w1020]
                tunnel: w1009 -> [w1015 w1019]
                tunnel: [w1016 w1018] -> w1007
                tunnel: [w1015 w1017] -> w1012
                frame False {
                }
                frame True {
                  n493 = stacked-sequence {
                    tunnel: w1020 -> [w1024 _]
                    tunnel: w1019 -> [w1023 _]
                    tunnel: [w1022 _] -> w1018
                    tunnel: [w1021 _] -> w1017
                    frame #0 {
                      # "ADQUISICIÓN"
                      n494 = flat-sequence {
                        tunnel: w1023 -> [w1043]
                        tunnel: w1024 -> [w1044]
                        tunnel: [w1054] -> w1034
                        tunnel: [w1053] -> w1033
                        tunnel: [w1052] -> w1032
                        tunnel: [w1051] -> w1031
                        tunnel: [w1050] -> w1030
                        tunnel: [w1049] -> w1029
                        tunnel: [w1071] -> w1028
                        tunnel: [w1070] -> w1027
                        tunnel: [w1069] -> w1026
                        tunnel: [w1062] -> w1025
                        tunnel: w1034 -> [w1068]
                        tunnel: w1033 -> [w1067]
                        tunnel: w1032 -> [w1066]
                        tunnel: w1031 -> [w1065]
                        tunnel: w1030 -> [w1064]
                        tunnel: w1029 -> [w1063]
                        tunnel: w1028 -> [w1138]
                        tunnel: w1027 -> [w1137]
                        tunnel: w1026 -> [w1140]
                        tunnel: w1025 -> [w1139]
                        tunnel: [w1141] -> w1021
                        tunnel: [w1142] -> w1022
                        frame #0 {
                          w1037 = T1 2 items=["51.200 kS/s (NI 9234)"=1, "25.600 kS/s (NI 9234)"=2, "17.067 kS/s (NI 9234)"=3, "12.800 kS/s (NI 9234)"=4, "10.240 kS/s (NI 9234)"=5, "8.533 kS/s (NI 9234)"=6, "7.314 kS/s (NI 9234)"=7, "6.400 kS/s (NI 9234)"=8, "5.689 kS/s (NI 9234)"=9, "5.120 kS/s (NI 9234)"=10, "4.654 kS/s (NI 9234)"=11, "4.267 kS/s (NI 9234)"=12, "3.938 kS/s (NI 9234)"=13, "3.657 kS/s (NI 9234)"=14, "3.413 kS/s (NI 9234)"=15, "3.200 kS/s (NI 9234)"=16, "3.012 kS/s (NI 9234)"=17, "2.845 kS/s (NI 9234)"=18, "2.695 kS/s (NI 9234)"=19, "2.560 kS/s (NI 9234)"=20, "2.438 kS/s (NI 9234)"=21, "2.328 kS/s (NI 9234)"=22, "2.226 kS/s (NI 9234)"=23, "2.133 kS/s (NI 9234)"=24, "2.048 kS/s (NI 9234)"=25, "1.969 kS/s (NI 9234)"=26, "1.896 kS/s (NI 9234)"=27, "1.829 kS/s (NI 9234)"=28, "1.765 kS/s (NI 9234)"=29, "1.707 kS/s (NI 9234)"=30, "1.652 kS/s (NI 9234)"=31] ("Data Rate")
                          n495 = xnode "Read/Write Control"("FPGA VI Reference In"=w1044, "error in"=w1043, "Fotocélula"=TRUE ("Adquirir")) -> ("FPGA VI Reference Out"=w1042:refnum<k20>, "error out"=w1041:errorcluster)
                          n496 = xnode "Read/Write Control"("FPGA VI Reference In"=w1042, "error in"=w1041, "Data Rate"=w1037, "Digital?"=TRUE, "Count(mSec)"=u32 2) -> ("FPGA VI Reference Out"=w1047:refnum<k20>, "error out"=w1046:errorcluster)
                          n497 = call "DMACalc.vi"("Number of Channels"=u32 10 ("Canales a calibrar (4 o 8)"), "Number of Samples"=u32 5000, "Rate (Hz)"=25600.0 ("Frecuencia de muestreo (Hz) 2")) -> ("Block Size"=w1051:u32, "Time to Acquire Block (ms)"=w1052:i32, "Host Buffer Size"=w1056:u32)  [unwired: 6 in]
                          n498 = call "Pathhorafech_calibration.vi"() -> ("path"=w1055:path)
                          "Nombre de archivo 2" <- w1055
                          n499 = xnode "Invoke Method"("FPGA VI Reference In"=w1047, "error in"=w1046, "Requested Depth"=w1056) -> ("FPGA VI Reference Out"=w1058:refnum<k20>, "error out"=w1057:errorcluster)  [unwired: 1 out]
                          n500 = Get Date/Time In Seconds() -> (seconds since 1Jan1904=→"Inicio pasada 2":timestamp)
                          n501 = xnode "Invoke Method"("FPGA VI Reference In"=w1058, "error in"=w1057) -> ("FPGA VI Reference Out"=w1054:refnum<k20>, "error out"=w1053:errorcluster)
                          n502 = Open/Create/Replace File(file path (use dialog)=w1055, operation (0:open)=T6."replace or create", access (0:read/write)=enum16{"read/write", "read-only", "write-only"}."read/write", disable buffering (F)=TRUE) -> (refnum out=w1050:refnum<file>, error out=w1049:errorcluster)  [unwired: 1 in, 2 out]
                        }
                        frame #1 {
                          n503 = while "Data Acquisition" {
                            tunnel: w1068 -> [w1097]
                            shift-right: [w1104] -> _
                            shift-left: u32 0 ("t") -> [w1100]
                            tunnel: w1066 -> [w1105]
                            tunnel: w1065 -> [w1103]
                            shift-right: [w1106] -> w1070
                            shift-left: w1067 -> [w1096]
                            tunnel: [w1101] -> w1071
                            tunnel: w1064 -> [w1084]
                            tunnel: [w1085] -> w1069
                            shift-right: [w1083] -> w1062
                            shift-left: w1063 -> [w1094]
                            stop <- w1102 stop-if-true
                            # "Detector de presencia"
                            # "Mide el tiempo de paso del tren y con ello se puede calcular\nla velocidad la unidad"
                            n504 = xnode "Invoke Method"("FPGA VI Reference In"=w1097, "error in"=w1096, "Number of Elements"=w1100, "Timeout (ms)"=0) -> ("FPGA VI Reference Out"=w1082:refnum<k20>, "error out"=w1081:errorcluster, "Data"=w1095:fxp<+/-,24,4>[], "Elements Remaining"=w1098:u32)
                            n505 = case "Data Ready" shown="Default" w1100 {
                              tunnel: w1105 -> [w1111 _]
                              tunnel: [w1110 u32 0 ("t")] -> w1104
                              tunnel: w1103 -> [w1112 _]
                              tunnel: w1098 -> [w1109 _]
                              tunnel: w1095 -> [_ w1122]
                              tunnel: w1094 -> [w1108 w1124]
                              tunnel: [w1108 w1123] -> w1083
                              tunnel: w1084 -> [w1107 w1121]
                              tunnel: [w1107 w1120] -> w1085
                              frame 0 {
                                # "En este caso se compara los elementos que quedan en la FIFO del controlador\ncon el tamaño dell bloque que aparece en el panel frontal. Si el número de\nelementos en la FIFO es mayor o igual que el tamaño del bloque se pasa al\nsiguiente caso y se guardan los datos en un archivo. El reloj que aparece es\nuna espera para no consumir recursos."
                                n506 = Greater Or Equal?(x=w1109, y=w1112) -> (x >= y?=w1113:bool)
                                n507 = case shown="True" w1113 {
                                tunnel: [u32 0 ("Block Size") w1117] -> w1110
                                tunnel: [w1116 0 ("t")] -> w1114
                                tunnel: w1111 -> [w1116 _]
                                tunnel: w1112 -> [_ w1117]
                                frame False {
                                }
                                frame True {
                                }
                                }
                                n508 = call "WaitMinTimeBetweenCall.vi"("Minimum ms between calls"=w1114) -> ()  [unwired: 2 in]
                              }
                              frame Default {
                                # "Se guardan los datos en el disco duro\nde Compact RIO"
                                n509 = To Single Precision Float(number=w1122) -> (single precision float=w1119:sgl[])
                                n510 = Write to Binary File(file (use dialog)=w1121, data=w1119, error in=w1124, 5:FALSE ("prepend array or string size? (T)"), 9:T7."little-endian" ("byte order (0:big-endian, network order)")) -> (refnum out=w1120:refnum<file>, error out=w1123:errorcluster)  [unwired: 2 out]
                              }
                            }
                            n511 = local read "Inicio pasada 2"() -> (w1079:timestamp)
                            n512 = Get Date/Time In Seconds() -> (seconds since 1Jan1904=w1078:timestamp)
                            n513 = To Double Precision Float(number=w1078) -> (double precision float=w1077:dbl)
                            n514 = To Double Precision Float(number=w1079) -> (double precision float=w1080:dbl)
                            n515 = Subtract(x=w1077, y=w1080) -> (x-y=w1087:dbl)
                            "Tiempo de paso (s) 2" <- w1087
                            n516 = xnode ("CheckLate")("FPGA VI Reference In"=w1082, "error in"=w1081) -> ("FPGA VI Reference Out"=w1074:refnum<k20>, "error out"=w1090:errorcluster, "Buffer Underflow"=w1091:bool, "Buffer Overflow"=w1092:bool)
                            "Buffer Underflow 2" <- w1091
                            "Buffer Overflow 2" <- w1092
                            n517 = Greater?(x=w1087, y=1.0 ("Tiempo de adquisición")) -> (0:w1076:bool)
                            n518 = call "ErrorOverFlow.vi"("Buffer Overflow"=w1092) -> ("error out"=w1088:errorcluster)
                            n519 = call "ErrorUnderFlow.vi"("Buffer Overflow"=w1091) -> ("error out"=w1089:errorcluster)
                            n520 = Merge Errors(w1090, w1089, w1088) -> (w1075:errorcluster)
                            n521 = Unbundle By Name(w1083) -> ("status"=w1086:bool)
                            n522 = Unbundle By Name(w1075) -> ("status"=w1093:bool)
                            n523 = Compound Arithmetic op=OR(w1093, w1076, w1086) -> (w1102:bool)
                            n524 = case "Flush" shown="True" w1102 {
                              tunnel: w1074 -> [w1128 w1133]
                              tunnel: w1075 -> [w1129 w1132]
                              tunnel: [w1129 w1131] -> w1106
                              tunnel: [w1128 w1130] -> w1101
                              frame False {
                              }
                              frame True {
                                n525 = xnode "Invoke Method"("FPGA VI Reference In"=w1133, "error in"=w1132) -> ("FPGA VI Reference Out"=w1130:refnum<k20>, "error out"=w1131:errorcluster)
                              }
                            }
                          }
                        }
                        frame #2 {
                          n526 = xnode "Read/Write Control"("FPGA VI Reference In"=w1138, "error in"=w1137, "Stop"=TRUE ("stop")) -> ("FPGA VI Reference Out"=w1136:refnum<k20>, "error out"=w1135:errorcluster)
                          n527 = Close File(refnum=w1140, error in=w1139) -> ()  [unwired: 2 out]
                          n528 = xnode "Invoke Method"("FPGA VI Reference In"=w1136, "error in"=w1135) -> ("FPGA VI Reference Out"=w1142:refnum<k20>, "error out"=w1141:errorcluster)
                        }
                      }
                    }
                    frame #1 {
                      # "PROCESADO"
                      n529 = local read "Nombre de archivo 2"() -> (w1167:path)
                      n530 = Read from Binary File(5:sgl 1.25, 9:T7."little-endian" ("byte order (0:big-endian, network order)"), 10:-1 ("count (1)"), 11:w1167) -> (0:w1170:errorcluster, 2:w1164:sgl[], 3:w1166:refnum<file>)  [unwired: 1 in, 2 out]
                      n531 = Close File(refnum=w1166, error in=w1170) -> ()  [unwired: 2 out]
                      n532 = Decimate 1D Array(w1164) -> (w1151:sgl[], w1152:sgl[], w1150:sgl[], w1146:sgl[], w1145:sgl[], w1147:sgl[], w1148:sgl[], w1149:sgl[], w1144:sgl[], w1143:sgl[])
                      n533 = Build Array(w1151, w1152, w1150, w1146, w1145, w1147, w1148, w1149, w1144, w1143) -> (w1163:sgl[][])
                      n534 = local read "Nº del canal"() -> (w1162:i32)
                      n535 = Delete From Array(array=w1163, index (row)=w1162) -> (deleted portion=w1156:sgl[])  [unwired: 2 in, 1 out]
                      n536 = stacked-sequence {
                        tunnel: [w1184] -> w1161
                        tunnel: [w1174] -> w1158
                        tunnel: w1156 -> [w1181]
                        tunnel: [w1172] -> w1153
                        frame #0 {
                          w1171 = 25600.0 ("Frecuencia de muestreo (Hz) 2")
                          # "1g=9,8m/s2"
                          n537 = Multiply(x="Parámetro de sensibilidad\n           (mV/g)", y=0.001) -> (x*y=w1186:dbl)
                          n538 = Divide(x=w1181, y=w1186) -> (x/y=w1180:dbl[])
                          n539 = call-poly <vilib>:"Basic Averaged DC-RMS.vi"("signal in"=w1180) -> ("DC value"=w1183:dbl)  [unwired: 7 in, 3 out]
                          n540 = Subtract(x=w1180, y=w1183) -> (x-y=w1173:dbl[])
                          n541 = Reciprocal(x=w1171) -> (1/x=w1174:dbl)
                          n542 = Divide(x=w1171, y="Frecuencia del patrón (Hz)") -> (x/y=w1177:dbl)
                          n543 = Array Size(array=w1173) -> (size(s)=w1178:i32)
                          n544 = Subtract(x=w1178, y=w1177) -> (x-y=w1179:dbl)
                          n545 = Bundle By Name("Y"=w1173, "dt"=w1174) -> (w1184:waveform(dbl))  [unwired: 1 in]
                          n546 = for {
                            N: w1179 -> [_]
                            tunnel: w1177 -> [w1193]
                            tunnel: [w1196] -> w1176 mode=indexing
                            tunnel: w1173 -> [w1195]
                            i -> [w1194]
                            n547 = Array Subset(array=w1195, index=w1194, length=w1193) -> (w1192:dbl[])
                            n548 = call-poly <vilib>:"RMS.vi"("X"=w1192) -> ("rms value"=w1196:dbl)  [unwired: 1 out]
                          }
                          n549 = call-poly <vilib>:"FFT Spectrum (Mag-Phase).vi"("time signal"=w1184) -> ("magnitude"=w1187:cluster{"f0":dbl, "df":dbl, "magnitude":dbl[]})  [unwired: 6 in, 4 out]
                          "Waveform Graph 3" <- w1187
                          n550 = Unbundle(w1187) -> ("df"=w1189:dbl, "magnitude"=w1190:dbl[])  [unwired: 1 out]
                          n551 = Array Max & Min(array=w1190) -> (max index (indices)=w1191:i32)  [unwired: 3 out]
                          n552 = Bundle By Name("Y"=w1176, "dt"=w1174) -> (w1172:waveform(dbl))  [unwired: 1 in]
                          n553 = Multiply(x=w1189, y=w1191) -> (x*y=→"Frecuencia de excitación\nVibrómetro  (Hz)":dbl)
                        }
                      }
                      n554 = Array Size(array=w1156) -> (size(s)=w1160:i32)
                      n555 = Initialize Array("Aceleración del patrón (g RMS)", w1160) -> (w1159:dbl[])
                      n556 = Bundle By Name("Y"=w1159, "dt"=w1158) -> (w1155:waveform(dbl))  [unwired: 1 in]
                      n557 = Build Array(w1161, w1153, w1155) -> (→"Waveform Graph 4":waveform(dbl)[])
                    }
                  }
                }
              }
              n558 = Wait (ms)(milliseconds to wait=u32 10) -> ()  [unwired: 1 out]
            }
          }
        }
        "error manipulacion archivos" <- w86
        "Estado" <- w81
        n559 = local read "Parar la aplicación"() -> (w84:bool)
      }
      n560 = xnode "Close FPGA VI Reference"("FPGA VI Reference In"=w76, "error in"=w75) -> ("error out"=→"error FPGA":errorcluster)
    }
    frame #3 {
      n561 = local read "RFID_ID"() -> (w1199:refnum<k5>)
      n562 = call "LH6HD.vi"("Action"=enum16{"Init", "Start", "Read", "Stop", "Exit"}."Stop") -> ("error out"=→"RFID_LR6_Error":errorcluster)  [unwired: 9 in, 1 out]
      n563 = TCP Close Connection(connection ID=w1199) -> (error out=→"RFID_Error":errorcluster)  [unwired: 1 in, 2 out]
    }
  }
